vi "NI32LV90ASD1_DAQLinescan.vi"() -> ()   [LabVIEW 2009]
uses:
  ImageSettings.ctt
  DisplaySettings.ctt
  Instance          51 19Saved   DAQLinescan .vi
  Instance          52 19Saved   DAQLinescan .vi
  <vilib>/Utility/inputDevices.llb/mouseAcquire.vi
panel:
  in  "Laser 5":bool
  in  "Laser 8":bool
  in  "Laser 7":bool
  in  "Laser 6":bool
  out "Position":dbl[](array[numeric]) format="%.6f"
  in  "show position (PI digital)":bool
  in  "mouse wheel\nfocus control":bool
  out "mouse focus":cluster{"device ID":refnum<k1>, "Scrolling":i32}
  in  "Laser 4":bool
  in  "SyncTime(ns)":dbl=12.5
  in  "Laser 3":bool
  in  "Laser 2":bool
  in  "Laser 1":bool
  in  "AOTF":u16(ring) items=["None", "Laser 1", "Laser 2", "Laser 1 + 2", "Laser 3", "Laser 1 + 3", "Laser 2 + 3", "Laser 1+2+3", "Laser 1+2+3+4", "Laser 2+3+4"]
  in  "AOTF Setup":bool
  in  "x-scale: Time?":bool
  in  "Autoscale y-axis":bool=TRUE
  in  "Store Data":bool
  in  "Pick & Destroy":bool caption="stop"
  in  "Load Image":bool caption="stop"
  in  "Position Increment (µm)":cluster{"x":dbl, "y":dbl, "z":dbl}={"x"=0.1, "y"=0.1, "z"=0.1} {"z" format="%.2f"; "y" format="%.2f"; "x" format="%.2f"}
  in  "Current Position (µm)":cluster{"x":dbl, "y":dbl, "z":dbl} {"z" format="%.2f"; "y" format="%.2f"; "x" format="%.2f"}
  in  "Down (z)":bool
  in  "Up (z)":bool
  in  "Down":bool
  in  "Up":bool
  in  "Right":bool
  in  "Left":bool
  in  "Display Settings":T1={"Show MCS"=TRUE, "Show Image"=TRUE, "Color coding"=1, "Plane"=0, "Threshold"={"max"=150, "min"=0}} {"Plane" max=0; "Color coding" items=["Color Gradient", "False Color"]}
  in  "Destination:":path
  in  "Exit":bool caption="stop"
  in  "Save & Exit":bool caption="stop"
  in  "Stage Setup":bool
  in  "SPC Setup":bool
  in  "Scan":bool
  in  "EOM Setup":bool
  in  "Keep Start Position":bool=TRUE
  in  "Isotropy (x/y)":bool=TRUE
  in  "Keep Image Size":bool=TRUE
  in  "EOM":u16(ring) items=["None", "Trace", "Retrace", "All"]
  in  "Read Position":bool
  in  "Image Settings":T2={"Start Position (µm)"={"x"=0.0, "y"=0.0, "z"=0.0}, "End Position (µm)"={"x"=10.0, "y"=10.0, "z"=10.0}, "Image Resolution (nm/pixel)"={"x"=50.0, "y"=50.0, "z"=100.0}, "Image Size (µm)"={"x"=10.0, "y"=10.0, "z"=0.0}, "Image Size (pixel)"={"x"=200, "y"=200, "z"=0}, "Time Resolution\n(ms/pixel)"=1.0, "1st Axis"=0, "2nd Axis"=1, "Retrace"=FALSE, "Estimated Time"="00:00:40"} {"2nd Axis" items=["x", "y", "z"]; "1st Axis" items=["x", "y", "z"]; "Time Resolution\n(ms/pixel)" format="%.2f"; "Image Resolution (nm/pixel)"."z" format="%.2f"; "Image Resolution (nm/pixel)"."y" format="%.2f"; "Image Resolution (nm/pixel)"."x" format="%.2f"; "Image Size (µm)"."z" format="%.2f"; "Image Size (µm)"."y" format="%.2f"; "Image Size (µm)"."x" format="%.2f"; "End Position (µm)"."z" format="%.2f"; "End Position (µm)"."y" format="%.2f"; "End Position (µm)"."x" format="%.2f"; "Start Position (µm)"."z" format="%.2f"; "Start Position (µm)"."y" format="%.2f"; "Start Position (µm)"."x" format="%.2f"}
  out "MCS Trace":u32[][](graph)=[[5, 9, 9, 4, 5, 7, 7, 7, 4, 6, 5, 11, 11, 6, 8, 9, 8, 5, 6, 8, 5, 5, 8, 5, 6, 5, 4, 9, 6, 13, 5, 5, 6, 9, 9, 11, 9, 7, 5, 9, 10, 7, 6, 4, 9, 7, 8, 6, 9, 4, 7, 9, 3, 4, 6, 8, 5, 6, 5, 4, 6, 11, 8, 5, 9, 5, 8, 7, 8, 8, 7, 3, 5, 14, 7, 12, 10, 7, 8, 8, 7, 5, 6, 6, 6, 9, 9, 7, 8, 7, 9, 3, 11, 4, 8, 7, 4, 4, 4, 5, 6, 6, 12, 5, 8, 7, 8, 7, 5, 8, 10, 10, 9, 5, 7, 8, 4, 6, 9, 6, 8, 9, 9, 9, 3, 7, 4, 10, 8, 11, 8, 6, 7, 4, 6, 4, 11, 9, 11, 7, 8, 4, 6, 9, 11, 8, 11, 7, 6, 4, 13, 9, 5, 4, 8, 5, 11, 5, 6, 6, 6, 3, 8, 8, 8, 11, 8, 6, 5, 7, 10, 7, 10, 12, 6, 9, 7, 4, 8, 8, 9, 7, 6, 6, 5, 8, 8, 3, 10, 5, 5, 7, 9, 8, 14, 6, 9, 5, 8, 7], [0, 0, 0, 0, 0, 0, 0, 0, 0, 0, 0, 0, 0, 0, 0, 0, 0, 0, 0, 0, 0, 0, 0, 0, 0, 0, 0, 0, 0, 0, 0, 0, 0, 0, 0, 0, 0, 0, 0, 0, 0, 0, 0, 0, 0, 0, 0, 0, 0, 0, 0, 0, 0, 0, 0, 0, 0, 0, 0, 0, 0, 0, 0, 0, 0, 0, 0, 0, 0, 0, 0, 0, 0, 0, 0, 0, 0, 0, 0, 0, 0, 0, 0, 0, 0, 0, 0, 0, 0, 0, 0, 0, 0, 0, 0, 0, 0, 0, 0, 0, 0, 0, 0, 0, 0, 0, 0, 0, 0, 0, 0, 0, 0, 0, 0, 0, 0, 0, 0, 0, 0, 0, 0, 0, 0, 0, 0, 0, 0, 0, 0, 0, 0, 0, 0, 0, 0, 0, 0, 0, 0, 0, 0, 0, 0, 0, 0, 0, 0, 0, 0, 0, 0, 0, 0, 0, 0, 0, 0, 0, 0, 0, 0, 0, 0, 0, 0, 0, 0, 0, 0, 0, 0, 0, 0, 0, 0, 0, 0, 0, 0, 0, 0, 0, 0, 0, 0, 0, 0, 0, 0, 0, 0, 0, 0, 0, 0, 0, 0, 0], [0, 0, 0, 0, 0, 0, 0, 0, 0, 0, 0, 0, 0, 0, 0, 0, 0, 0, 0, 0, 0, 0, 0, 0, 0, 0, 0, 0, 0, 0, 0, 0, 0, 0, 0, 0, 0, 0, 0, 0, 0, 0, 0, 0, 0, 0, 0, 0, 0, 0, 0, 0, 0, 0, 0, 0, 0, 0, 0, 0, 0, 0, 0, 0, 0, 0, 0, 0, 0, 0, 0, 0, 0, 0, 0, 0, 0, 0, 0, 0, 0, 0, 0, 0, 0, 0, 0, 0, 0, 0, 0, 0, 0, 0, 0, 0, 0, 0, 0, 0, 0, 0, 0, 0, 0, 0, 0, 0, 0, 0, 0, 0, 0, 0, 0, 0, 0, 0, 0, 0, 0, 0, 0, 0, 0, 0, 0, 0, 0, 0, 0, 0, 0, 0, 0, 0, 0, 0, 0, 0, 0, 0, 0, 0, 0, 0, 0, 0, 0, 0, 0, 0, 0, 0, 0, 0, 0, 0, 0, 0, 0, 0, 0, 0, 0, 0, 0, 0, 0, 0, 0, 0, 0, 0, 0, 0, 0, 0, 0, 0, 0, 0, 0, 0, 0, 0, 0, 0, 0, 0, 0, 0, 0, 0, 0, 0, 0, 0, 0, 0]]
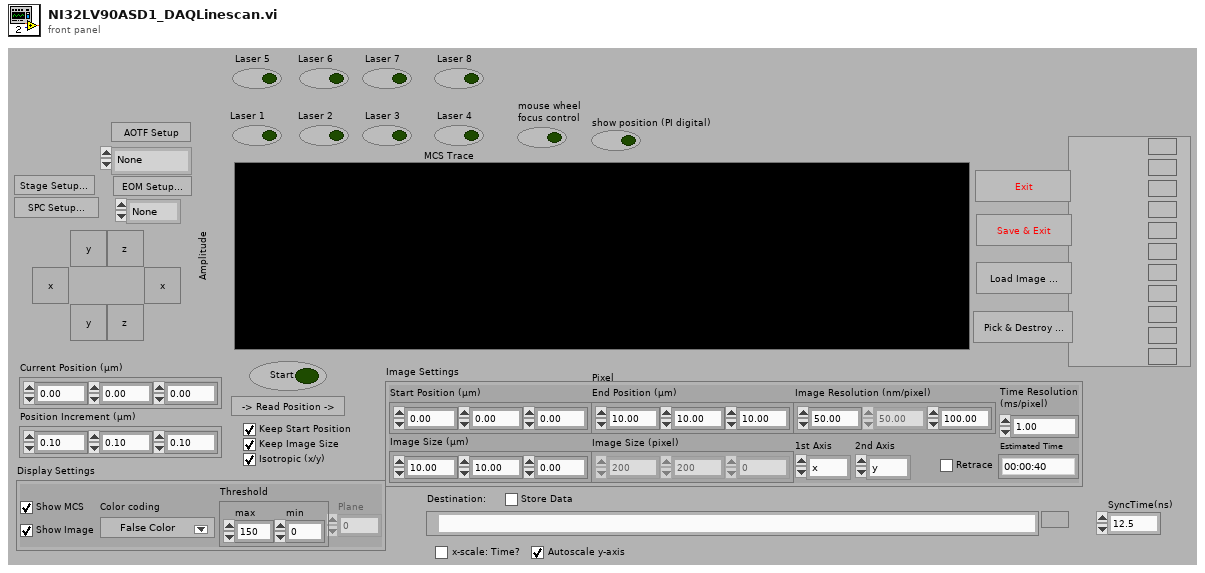
[diagram p1: front panel]
types:
  T1 = typedef "DisplaySettings.ctt" = cluster{"Show MCS":bool, "Show Image":bool, "Color coding":u16, "Plane":u32, "Threshold":cluster{"max":u32, "min":u32}}
  T2 = typedef "ImageSettings.ctt" = cluster{"Start Position (µm)":cluster{"x":dbl, "y":dbl, "z":dbl}, "End Position (µm)":cluster{"x":dbl, "y":dbl, "z":dbl}, "Image Resolution (nm/pixel)":cluster{"x":dbl, "y":dbl, "z":dbl}, "Image Size (µm)":cluster{"x":dbl, "y":dbl, "z":dbl}, "Image Size (pixel)":cluster{"x":u32, "y":u32, "z":u32}, "Time Resolution\n(ms/pixel)":dbl, "1st Axis":u16, "2nd Axis":u16, "Retrace":bool, "Estimated Time":string}
  T3 = enum16{"Get Type", "Set Type", "GetStageInit", "GetWriteStageSetting", "GetInitializeStageOutput", "GetSetAxisPosition", "GetSetPos", "GetSetupStage", "HaltStageOutput"}
  T4 = enum16{"Get Type", "Set Type", "GetStageInit", "GetWriteStageSetting", "GetInitializeStageOutput", "GetSetAxisPosition", "GetSetPos"}
  T5 = typedef "FIFOSettings.ctt" = cluster{"Measurement":cluster{"Binning (ms)":sgl, "External Trigger Condition":u16, "Stop Condition:":u16, "Stop Count":dbl, "Buffer Size (Photons)":u32, "No of Channels":u16, "Ext Latch Delay":i16}, "ADC":cluster{"Binning (HH)":i16, "Dither Range":i16, "Count Increment":i16, "Mode":u16}, "SYNC":cluster{"SYNC ZC Level (mV)":sgl, "SYNC Freq Divider":u16, "SYNC Holdoff (ps)":sgl, "SYNC Threshold (mV)":sgl}, "TAC":cluster{"TAC Range (ns)":sgl, "TAC Gain":i16, "TAC Offset (%)":sgl, "TAC Limit Low (%)":sgl, "TAC Limit High (%)":sgl}, "Ch 2":cluster{"Ch2 ZC Level (mV)":sgl, "Ch2 Holdoff (ps)":sgl, "Ch2 Threshold (mV)":sgl}, "Ch 3":cluster{"Ch3 ZC Level (mV)":sgl, "Ch3 Holdoff (ps)":sgl, "Ch3 Threshold (mV)":sgl}, "Ch 4":cluster{"Ch4 ZC Level (mV)":sgl, "Ch4 Holdoff (ps)":sgl, "Ch4 Threshold (mV)":sgl}, "Ch1":cluster{"Ch1 ZC Level (mV)":sgl, "Ch1 Holdoff (ps)":sgl, "Ch1 Threshold (mV)":sgl}}
  T6 = typedef "DAQLinescanVisualization.ctt" = cluster{"Threshold":u32, "Trace Window #":u32, "IMAQ Trace":T7, "Retrace Window #":u32, "IMAQ Retrace":T7}
  T7 = typedef "IMAQ Image.ctl" = refnum<image>
  T8 = typedef "LineScanStatus.ctt" = cluster{"in line":bool, "line status":cluster{"count":u32, "current":cluster{"x":u32, "y":u32, "z":u32}}, "plane status":cluster{"count":u32, "current":cluster{"x":u32, "y":u32, "z":u32}}, "new line step":cluster{"x":dbl, "y":dbl, "z":dbl}, "new plane step":cluster{"x":dbl, "y":dbl, "z":dbl}}
  T9 = typedef "StageType.ctt" = enum16{"PI 725 USB", "PI 725 TCP/IP", "PI analogue step"}
  T10 = cluster{"Start Position (µm)":cluster{"x":dbl, "y":dbl, "z":dbl}, "End Position (µm)":cluster{"x":dbl, "y":dbl, "z":dbl}, "Image Resolution (nm/pixel)":cluster{"x":dbl, "y":dbl, "z":dbl}, "Image Size (µm)":cluster{"x":dbl, "y":dbl, "z":dbl}, "Image Size (pixel)":cluster{"x":u32, "y":u32, "z":u32}, "Time Resolution\n(ms/pixel)":dbl, "1st Axis":u16, "2nd Axis":u16, "Retrace":bool, "Estimated Time":string}
  T11 = typedef "ScannedImage.ctl" = cluster{"BinningMicroS":dbl, "OverflowConstant":dbl, "MacrotimeCycle":dbl, "Trace":u32[][][][], "Retrace":u32[][][][], "current line":i32, "current plane":i32}
  T12 = cluster{"Horizontal":i32, "Vertical":i32, "Scrolling":i32}
  T13 = typedef "LVMinMaxIncTypeDef.ctl" = cluster{"Minimum":dbl, "Maximum":dbl, "Increment":dbl}
  T14 = typedef "AnalogSettings.ctt" = cluster{"PCI 671x Device Number":u32, "Samples per Unit":u32}
  T15 = typedef "AOTFSettings.ctt" = cluster{"Laser 1 Output Channel":tag, "AOTF  1 Output Voltage":dbl, "Laser 2 Output Channel":tag, "AOTF  2 Output Voltage":dbl, "Laser 3 Output Channel":tag, "AOTF  3 Output Voltage":dbl, "Pixel per Cycle":u16, "Time per Cycle  / ms":dbl, "Laser 4 Output Channel":tag, "AOTF  4 Output Voltage":dbl, "Laser 5 Output Channel":tag, "AOTF 5 Output Voltage ":dbl, "Laser 6 Output Channel":tag, "AOTF  6 Output Voltage ":dbl, "Laser 7 Output Channel":tag, "AOTF 7 Output Voltage ":dbl, "Laser 8 Output Channel":tag, "AOTF  8 Output Voltage ":dbl, "AOTF  1 Frequency":dbl, "AOTF  2 Frequency":dbl, "AOTF  3  Frequency":dbl, "AOTF  4 Frequency":dbl, "AOTF 5 Frequency":dbl, "AOTF  6 Frequency":dbl, "AOTF 7  Frequency":dbl, "AOTF  8 Frequency":dbl, "AOTF  1 Amplitude":dbl, "AOTF  2 Amplitude":dbl, "AOTF  3  Amplitude":dbl, "AOTF  4 Amplitude":dbl, "AOTF 5 Amplitude":dbl, "AOTF  6 Amplitude":dbl, "AOTF 7 Amplitude  ":dbl, "AOTF  8 Amplitude":dbl}
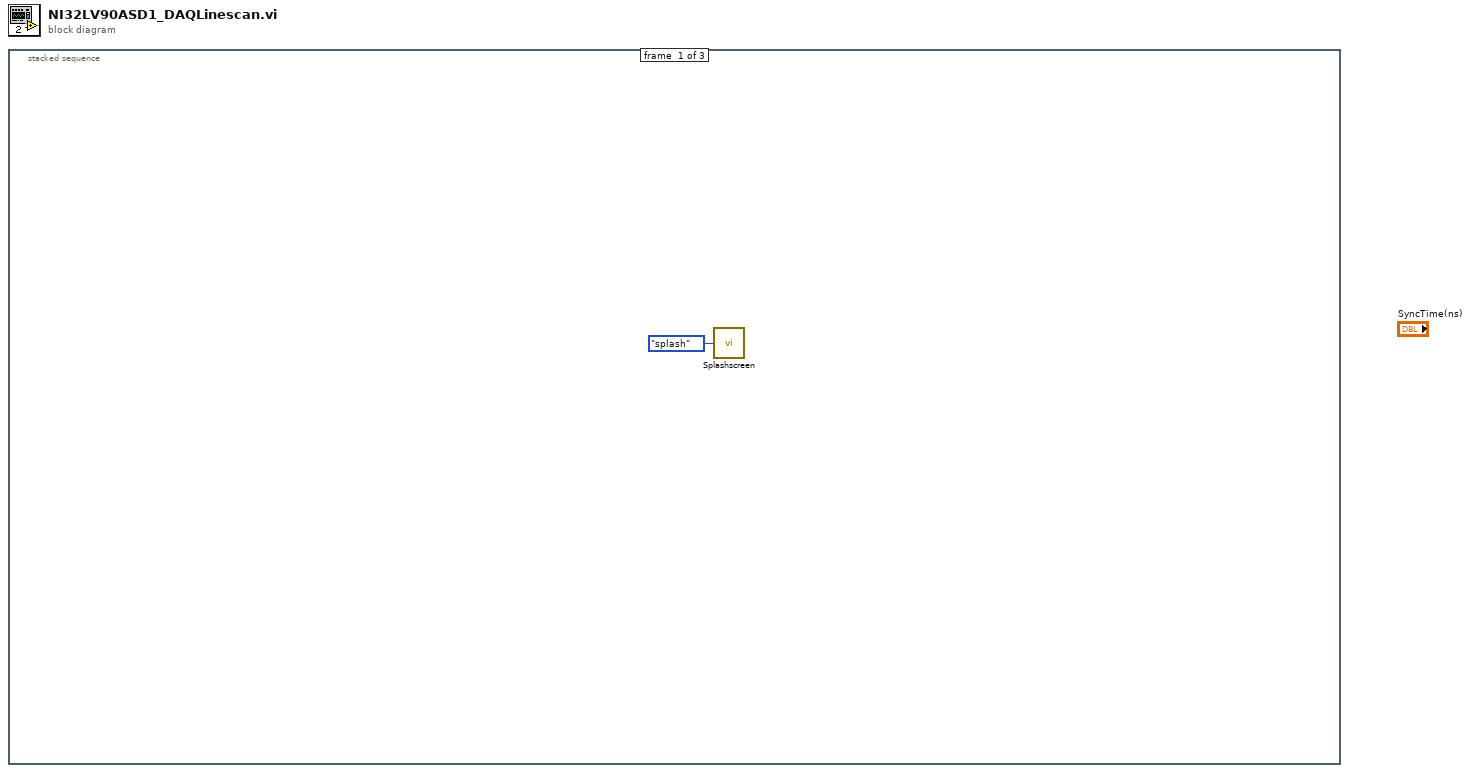
[diagram p0: block diagram]
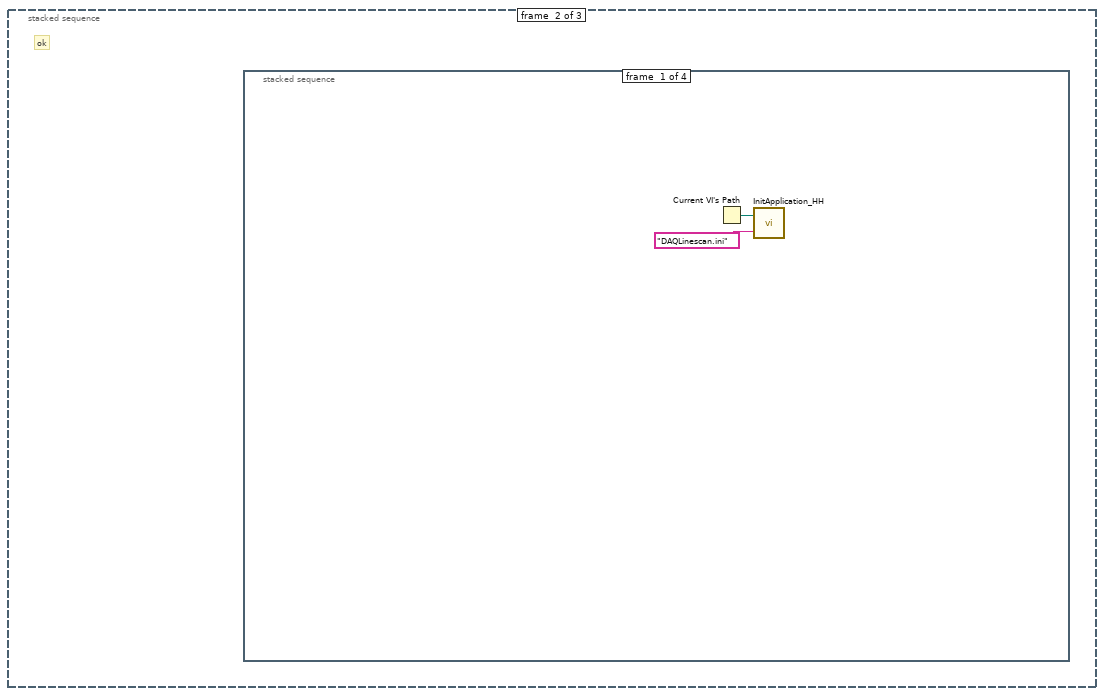
[diagram p2: hidden frame]
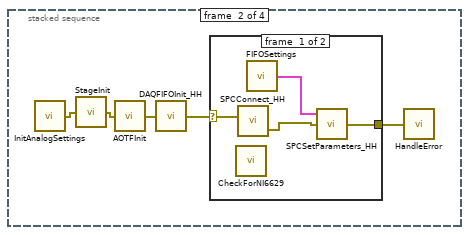
[diagram p3: hidden frame]
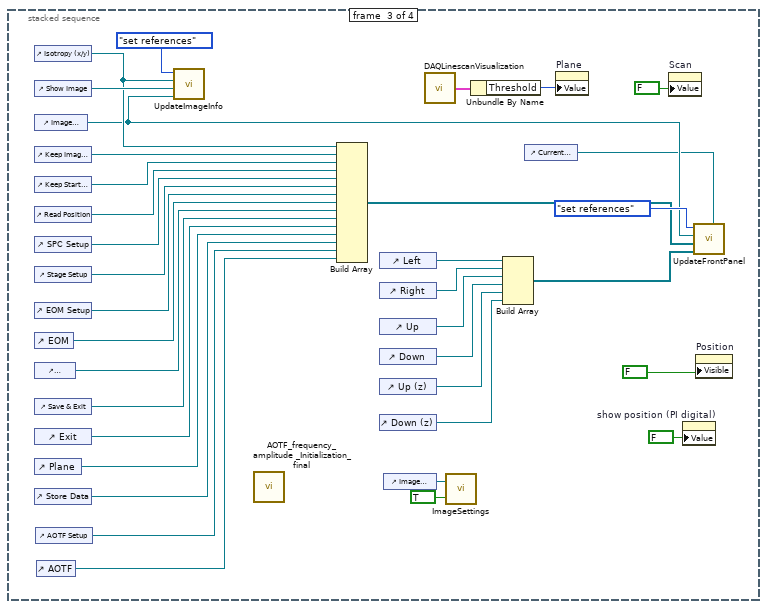
[diagram p5: hidden frame]
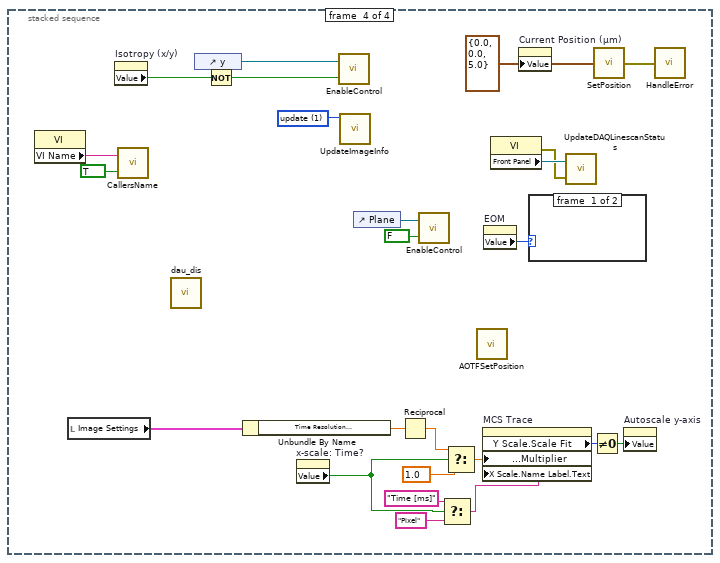
[diagram p6: hidden frame]
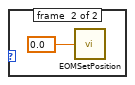
[diagram p7: hidden frame]
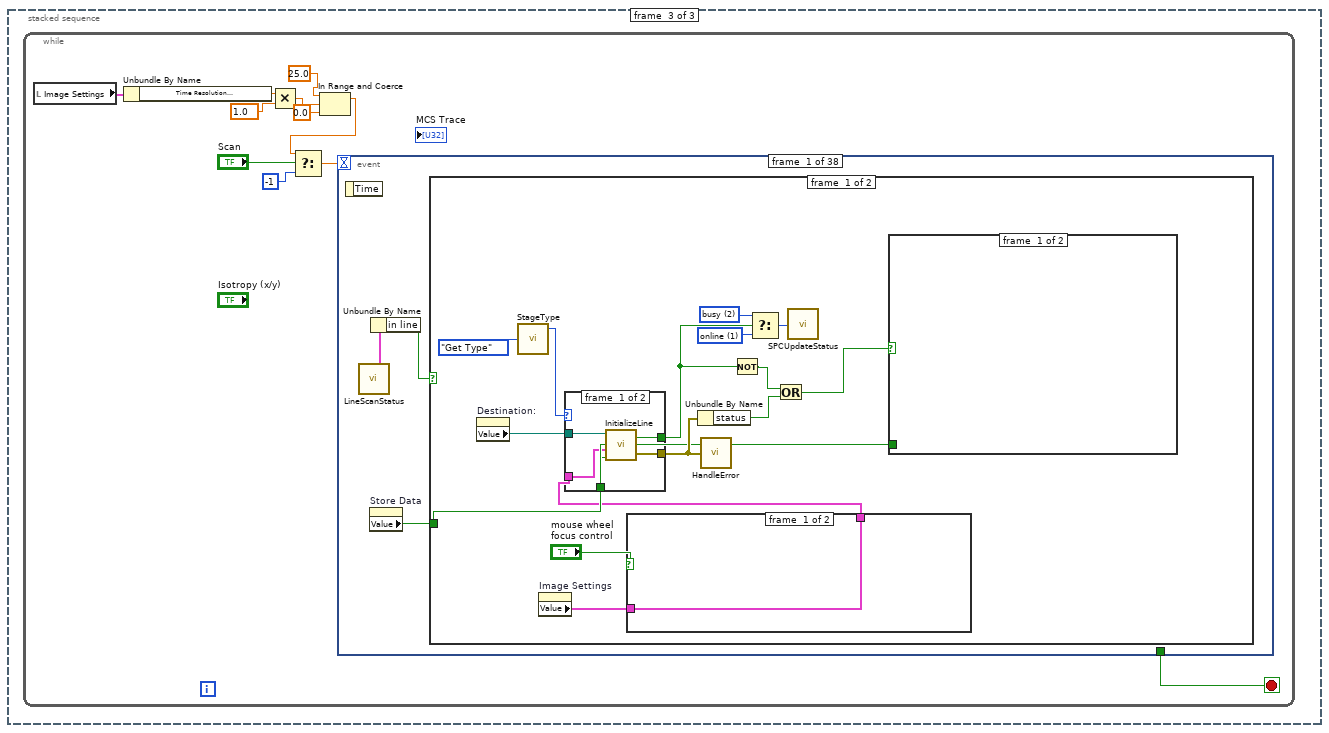
[diagram p8: hidden frame]
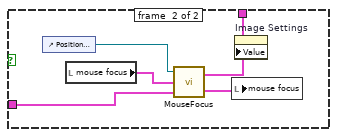
[diagram p9: hidden frame]
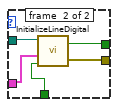
[diagram p10: hidden frame]
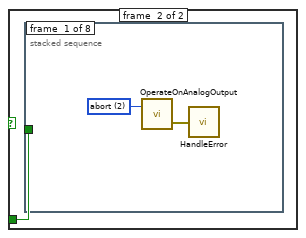
[diagram p11: hidden frame]
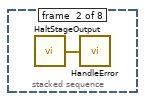
[diagram p12: hidden frame]
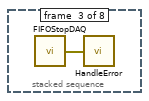
[diagram p13: hidden frame]
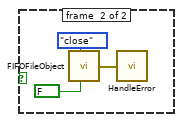
[diagram p15: hidden frame]
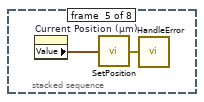
[diagram p16: hidden frame]
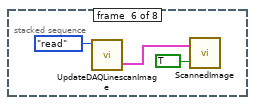
[diagram p17: hidden frame]
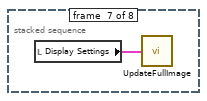
[diagram p18: hidden frame]
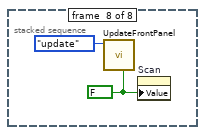
[diagram p19: hidden frame]
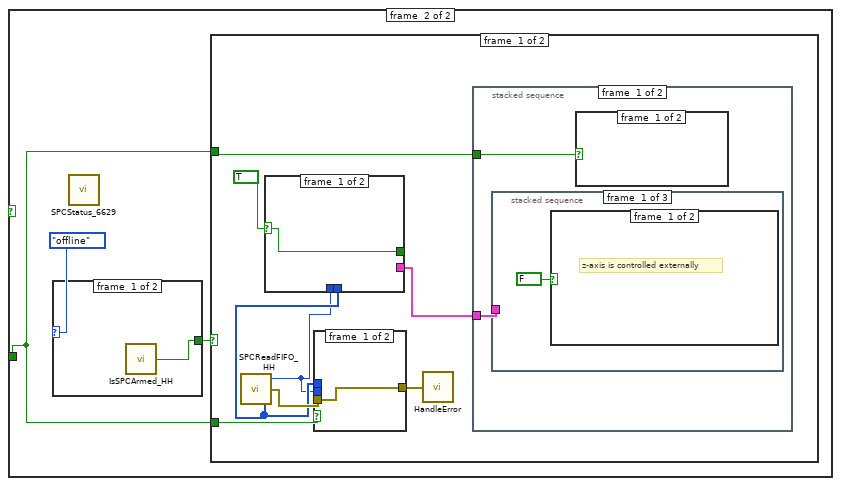
[diagram p20: hidden frame]
diagram:
  n1 = stacked-sequence {
    frame #0 {
      n2 = call "Splashscreen.vi"("Mode"=enum16{"splash", "dialog"}."splash") -> ()  [unwired: 1 in]
    }
    frame #1 {
      # "ok"
      n3 = stacked-sequence {
        frame #0 {
          n4 = Current VI's Path() -> (path=w3:path)
          n5 = call "InitApplication_HH.vi"("file name"="DAQLinescan.ini", "VI path"=w3) -> ()
        }
        frame #1 {
          n6 = call "InitAnalogSettings.vi"() -> ("error out"=w5:errorcluster)  [unwired: 1 in]
          n7 = call "StageInit.vi"("error in (no error)"=w5) -> ("error out"=w4:errorcluster)
          n8 = call "AOTFInit.vi"("error in (no error)"=w4) -> ("error out"=w6:errorcluster)
          n9 = call "DAQFIFOInit_HH.vi"("error in (no error)"=w6) -> ("error out"=w8:errorcluster)
          n10 = case shown="No Error" w8 {
            selector: w8 -> [w10 w13]
            tunnel: [w11 w13] -> w7
            frame #0 {
              n11 = call "CheckForNI6629.vi"() -> ()  [unwired: 1 in]
              n12 = call "SPCConnect_HH.vi"("error in (no error)"=w10) -> ("Error out"=w9:errorcluster)  [unwired: 1 in]
              n13 = call "FIFOSettings.vi"() -> ("FIFO Settings(out)"=w12:T5)  [unwired: 2 in]
              n14 = call "SPCSetParameters_HH.vi"("error in (no error)"=w9, "FIFO Settings"=w12) -> ("error (out)"=w11:errorcluster)  [unwired: 1 in]
            }
            frame #1 {
            }
          }
          n15 = call "HandleError.vi"("error in (no error)"=w7) -> ()
        }
        frame #2 {
          n16 = control-ref of="Isotropy (x/y)"() -> (w27:refnum<vi>)
          n17 = control-ref of="Show Image"() -> (w46:refnum<vi>)
          n18 = control-ref of="Image Settings"() -> (w26:refnum<vi>)
          n19 = control-ref of="Keep Image Size"() -> (w45:refnum<vi>)
          n20 = control-ref of="Keep Start Position"() -> (w44:refnum<vi>)
          n21 = control-ref of="Read Position"() -> (w43:refnum<vi>)
          n22 = control-ref of="SPC Setup"() -> (w42:refnum<vi>)
          n23 = control-ref of="Stage Setup"() -> (w41:refnum<vi>)
          n24 = control-ref of="EOM Setup"() -> (w40:refnum<vi>)
          n25 = control-ref of="EOM"() -> (w39:refnum<vi>)
          n26 = control-ref of="Destination:"() -> (w38:refnum<vi>)
          n27 = control-ref of="Save & Exit"() -> (w37:refnum<vi>)
          n28 = control-ref of="Exit"() -> (w36:refnum<vi>)
          n29 = control-ref of="Plane"() -> (w22:refnum<vi>)
          n30 = control-ref of="Store Data"() -> (w21:refnum<vi>)
          n31 = control-ref of="AOTF Setup"() -> (w17:refnum<vi>)
          n32 = control-ref of="AOTF"() -> (w16:refnum<vi>)
          n33 = call "UpdateImageInfo.vi"("Image Refnum"=w26, "Show Image Refnum"=w46, "Isotropy (x/y) Refnum"=w27, "operation"=enum16{"set references", "update"}."set references") -> ()
          n34 = call "AOTF_frequency_amplitude _Initialization_final.vi"() -> ()  [unwired: 1 in]
          n35 = Build Array(w27, w45, w44, w43, w42, w41, w40, w39, w38, w37, w36, w22, w21, w17, w16) -> (w25:refnum<vi>[])
          n36 = control-ref of="Left"() -> (w35:refnum<vi>)
          n37 = control-ref of="Right"() -> (w34:refnum<vi>)
          n38 = control-ref of="Up"() -> (w33:refnum<vi>)
          n39 = control-ref of="Down"() -> (w32:refnum<vi>)
          n40 = control-ref of="Up (z)"() -> (w31:refnum<vi>)
          n41 = control-ref of="Down (z)"() -> (w30:refnum<vi>)
          n42 = control-ref of="Image Settings"() -> (w19:refnum<vi>)
          n43 = call "DAQLinescanVisualization.vi"() -> ("Visualization (output)"=w47:T6)  [unwired: 2 in]
          n44 = call "ImageSettings.vi"("set"=TRUE ("s"), "Image Settings in"=w19) -> ()  [unwired: 1 out]
          n45 = Unbundle By Name(w47) -> ("Threshold"=w48:u32)
          n46 = Build Array(w35, w34, w33, w32, w31, w30) -> (w24:refnum<vi>[])
          n47 = control-ref of="Current Position (µm)"() -> (w23:refnum<vi>)
          n48 = property on="Plane" class="DigNum (strict)"("Value"=w48) -> ()  [unwired: 2 in, 2 out]
          n49 = property on="Scan" class="Bool (strict)"("Value"=FALSE ("Scan")) -> ()  [unwired: 2 in, 2 out]
          n50 = property on="show position (PI digital)" class="Bool (strict)"("Value"=FALSE ("show position (PI digital)")) -> ()  [unwired: 2 in, 2 out]
          n51 = call "UpdateFrontPanel.vi"("operation"=enum16{"set references", "update"}."set references", "Image Settings"=w26, "Regular Controls"=w25, "Special Controls"=w24, "Current Position (µm)"=w23) -> ()  [unwired: 5 in]
          n52 = property on="Position" class="Arr (strict)"("Visible"=FALSE) -> ()  [unwired: 2 in, 2 out]
        }
        frame #3 {
          w66 = u16 1 items=["set references", "update"] ("operation")
          w70 = cluster{"x":dbl, "y":dbl, "z":dbl} {"x"=0.0, "y"=0.0, "z"=5.0} ("Current Position (µm)")
          n53 = property class="VI"() -> ("VI Name"=w61:string)  [unwired: 2 in, 2 out]
          n54 = local read "Image Settings"() -> (w57:T2)
          n55 = property on="Isotropy (x/y)" class="Boolean (strict)"() -> ("Value"=w67:bool)  [unwired: 2 in, 2 out]
          n56 = call "CallersName.vi"("Get/Set"=TRUE ("s"), "Callers Name"=w61) -> ()  [unwired: 1 out]
          n57 = call "dau_dis.vi"() -> ()  [unwired: 1 in]
          n58 = control-ref of="y"() -> (w72:refnum<vi>)
          n59 = Not(x=w67) -> (.not. x?=w71:bool)
          n60 = Unbundle By Name(w57) -> ("Time Resolution\n(ms/pixel)"=w56:dbl)
          n61 = property on="x-scale: Time?" class="Boolean (strict)"() -> ("Value"=w50:bool)  [unwired: 2 in, 2 out]
          n62 = call "EnableControl.vi"("Enable"=w71, "Reference"=w72) -> ()
          n63 = call "UpdateImageInfo.vi"("operation"=w66) -> ()  [unwired: 3 in]
          n64 = control-ref of="Plane"() -> (w65:refnum<vi>)
          n65 = Reciprocal(x=w56) -> (1/x=w54:dbl)
          n66 = call "EnableControl.vi"("Enable"=FALSE, "Reference"=w65) -> ()
          n67 = Select(t="Time [ms]", s=w50, f="Pixel") -> (s? t:f=w49:string)
          n68 = Select(t=w54, s=w50, f=1.0) -> (s? t:f=w55:dbl)
          n69 = call "AOTFSetPosition.vi"() -> ()  [unwired: 2 in]
          n70 = property on="MCS Trace" class="WaveformChart (strict)"("X Scale.Offset and Multiplier:Multiplier"=w55, "X Scale.Name Label.Text"=w49) -> ("Y Scale.Scale Fit"=w59:u8)  [unwired: 2 in, 2 out]
          n71 = property on="EOM" class="Ring (strict)"() -> ("Value"=w62:u16)  [unwired: 2 in, 2 out]
          n72 = property class="VI"() -> (error out=w68:errorcluster, "Front Panel"=w69:refnum<vi>)  [unwired: 2 in, 1 out]
          n73 = property on="Current Position (µm)" class="Cluster (strict)"("Value"=w70) -> ()  [unwired: 2 in, 2 out]
          n74 = case shown="0" w62 {
            frame #0 {
            }
            frame #1 {
              n75 = call "EOMSetPosition.vi"("value"=sgl 0.0) -> ()
            }
          }
          n76 = call "UpdateDAQLinescanStatus.vi"("error in (no error)"=w68, "Panel"=w69) -> ()
          n77 = Not Equal To 0?(x=w59) -> (x != 0?=w58:bool)
          n78 = call "SetPosition.vi"("Current Position (µm)"=w70) -> ("error out"=w63:errorcluster)
          n79 = property on="Autoscale y-axis" class="Bool (strict)"("Value"=w58) -> ()  [unwired: 2 in, 2 out]
          n80 = call "HandleError.vi"("error in (no error)"=w63) -> ()
        }
      }
    }
    frame #2 {
      n81 = while {
        stop <- w80 stop-if-true
        n82 = local read "Image Settings"() -> (w81:T2)
        n83 = Unbundle By Name(w81) -> ("Time Resolution\n(ms/pixel)"=w79:dbl)
        n84 = Multiply(x=w79, y=1.0) -> (x*y=w77:dbl)
        n85 = In Range and Coerce(upper limit=25.0, x=w77, lower limit=0.0) -> (coerced(x)=w74:dbl)  [unwired: 1 out]
        n86 = Select(t=w74, s="Scan", f=-1) -> (s? t:f=w84:dbl)
        n87 = event shown="[28] \"Pick & Destroy\": Value Change" {
          selector: _ -> [_ _ _ _ _ _ _ _ _ _ _ _ _ _ _ _ _ _ _ _ _ _ _ _ _ _ _ _ _ _ _ _ _ _ _ _ _ _]
          dyn-events: _ -> [_ _ _ _ _ _ _ _ _ _ _ _ _ _ _ _ _ _ _ _ _ _ _ _ _ _ _ _ _ _ _ _ _ _ _ _ _ _]
          timeout: w84 -> [_ _ _ _ _ _ _ _ _ _ _ _ _ _ _ _ _ _ _ _ _ _ _ _ _ _ _ _ _ _ _ _ _ _ _ _ _ _]
          tunnel: [_ _ _ _ _ _ _ _ _ _ _ _ _ _ _ _ _ _ _ _ _ _ _ _ _ TRUE _ _ _ _ _ _ _ _ _ _ _ _] -> w80
          event #0 {
            n88 = event-data() -> ()  [unwired: 1 in, 1 out]
            n89 = call "LineScanStatus.vi"() -> ("Linescan Status (output)"=w86:T8)  [unwired: 2 in]
            n90 = property on="Store Data" class="Boolean (strict)"() -> ("Value"=w85:bool)  [unwired: 2 in, 2 out]
            n91 = Unbundle By Name(w86) -> ("in line"=w87:bool)
            n92 = case shown="True" w87 {
              tunnel: w85 -> [w93 w138]
              frame #0 {
                w100 = u16 1 items=["offline", "online", "busy"] ("Status (input)")
                w101 = u16 2 items=["offline", "online", "busy"] ("Status (input)")
                n93 = property on="Destination:" class="Path"() -> ("Value"=w102:path)  [unwired: 2 in, 2 out]
                n94 = call "StageType.vi"("Function"=T3."Get Type") -> ("Stage Type (output)"=w91:T9)  [unwired: 2 in, 2 out]
                n95 = property on="Image Settings" class="Cluster (strict)"() -> ("Value"=w90:T10)  [unwired: 2 in, 2 out]
                n96 = case shown="False" "mouse wheel\nfocus control" {
                  tunnel: w90 -> [w103 w108]
                  tunnel: [w103 w107] -> w89
                  frame #0 {
                  }
                  frame #1 {
                    n97 = control-ref of="Position Increment (µm)"() -> (w104:refnum<vi>)
                    n98 = local read "mouse focus"() -> (w106:cluster{"device ID":refnum<k1>, "Scrolling":i32})
                    n99 = call "MouseFocus.vi"("Image Settings"=w108, "mouse focus"=w106, "Position increment"=w104) -> ("mouse focus"=w105:cluster{"device ID":refnum<k1>, "Scrolling":i32}, "Image Settings"=w107:T10)
                    n100 = local write "mouse focus"(w105) -> ()
                    n101 = property on="Image Settings" class="Clust (strict)"("Value"=w107) -> ()  [unwired: 2 in, 2 out]
                  }
                }
                n102 = case shown="\"PI 725 USB\", \"PI 725 TCP/IP\"" w91 {
                  tunnel: w102 -> [w113 w118]
                  tunnel: w89 -> [w112 w117]
                  tunnel: [w111 w115] -> w98
                  tunnel: [w110 w114] -> w97
                  tunnel: w93 -> [w109 w116]
                  frame #0 {
                    n103 = call "InitializeLine.vi"("Store Data"=w109, "Image Settings"=w112, "Destination:"=w113) -> ("error out"=w111:errorcluster, "Busy"=w110:bool)  [unwired: 1 in]
                  }
                  frame #1 {
                    n104 = call "InitializeLineDigital.vi"("Store Data"=w116, "Image Settings"=w117, "Destination:"=w118) -> ("error out"=w115:errorcluster, "Busy"=w114:bool)  [unwired: 1 in]
                  }
                }
                n105 = Unbundle By Name(w98) -> ("status"=w95:bool)
                n106 = call "HandleError.vi"("error in (no error)"=w98) -> ()
                n107 = Not(x=w97) -> (.not. x?=w96:bool)
                n108 = Select(t=w101, s=w97, f=w100) -> (s? t:f=w99:u16)
                n109 = Or(x=w96, y=w95) -> (x .or. y?=w94:bool)
                n110 = call "SPCUpdateStatus.vi"("Status"=w99) -> ()
                n111 = case shown="True" w94 {
                  tunnel: w93 -> [_ w119]
                  frame #0 {
                  }
                  frame #1 {
                    n112 = stacked-sequence {
                      tunnel: w119 -> [_ _ _ w124 _ _ _ _]
                      frame #0 {
                        w121 = u16 2 items=["start", "state", "abort"] ("operation")
                        n113 = call "OperateOnAnalogOutput.vi"("operation"=w121) -> ("error out"=w120:errorcluster)  [unwired: 1 in, 1 out]
                        n114 = call "HandleError.vi"("error in (no error)"=w120) -> ()
                      }
                      frame #1 {
                        n115 = call "HaltStageOutput.vi"() -> ("Error out"=w122:errorcluster)  [unwired: 1 in]
                        n116 = call "HandleError.vi"("error in (no error)"=w122) -> ()
                      }
                      frame #2 {
                        n117 = call "FIFOStopDAQ.vi"() -> ("error out"=w123:errorcluster)
                        n118 = call "HandleError.vi"("error in (no error)"=w123) -> ()
                      }
                      frame #3 {
                        n119 = case shown="True" w124 {
                          frame #0 {
                          }
                          frame #1 {
                            n120 = call "FIFOFileObject.vi"(".sm file format"=FALSE, "function (open:0)"=enum16{"open", "write", "close"}."close") -> ("error out"=w126:errorcluster)  [unwired: 4 in]
                            n121 = call "HandleError.vi"("error in (no error)"=w126) -> ()
                          }
                        }
                      }
                      frame #4 {
                        n122 = property on="Current Position (µm)" class="Cluster (strict)"() -> ("Value"=w129:cluster{"x":dbl, "y":dbl, "z":dbl})  [unwired: 2 in, 2 out]
                        n123 = call "SetPosition.vi"("Current Position (µm)"=w129) -> ("error out"=w128:errorcluster)
                        n124 = call "HandleError.vi"("error in (no error)"=w128) -> ()
                      }
                      frame #5 {
                        n125 = call "UpdateDAQLinescanImage.vi"("operation"=enum16{"initialize", "update", "read"}."read") -> ("LinescanSampling"=w132:T11)  [unwired: 3 in, 1 out]
                        n126 = call "ScannedImage.vi"("Get/Set"=TRUE, "Scanned Image (input)"=w132) -> ()  [unwired: 1 out]
                      }
                      frame #6 {
                        n127 = local read "Display Settings"() -> (w133:T1)
                        n128 = call "UpdateFullImage.vi"("Display Settings"=w133) -> ()
                      }
                      frame #7 {
                        w135 = FALSE ("Scan")
                        n129 = call "UpdateFrontPanel.vi"("operation"=enum16{"set references", "update"}."update", "Scan"=w135) -> ()  [unwired: 8 in]
                        n130 = property on="Scan" class="Boolean (strict)"("Value"=w135) -> ()  [unwired: 2 in, 2 out]
                      }
                    }
                  }
                }
              }
              frame #1 {
                n131 = case shown="\"offline\", Default" enum16{"offline", "online", "busy"}."offline" ("Status (output)") {
                  tunnel: [w139 FALSE] -> w137
                  frame #0 {
                    n132 = call "IsSPCArmed_HH.vi"() -> ("Boolean"=w139:bool)  [unwired: 1 in]
                  }
                  frame #1 {
                  }
                }
                n133 = call "SPCStatus_6629.vi"() -> ()  [unwired: 2 in, 1 out]
                n134 = case shown="True" w137 {
                  tunnel: w138 -> [w141 w186]
                  tunnel: w138 -> [w143 w185]
                  frame #0 {
                    n135 = call "SPCReadFIFO_HH.vi"() -> ("count"=w144:i32, "error out"=w148:errorcluster, "buffer"=w146:u32[])  [unwired: 2 in]
                    n136 = case shown="True" TRUE ("Case Constant\n(See Context Help) 2") {
                      selector: TRUE ("Case Constant\n(See Context Help) 2") -> [w169 _]
                      tunnel: w144 -> [_ w174]
                      tunnel: w146 -> [_ w173]
                      tunnel: [w169 w172] -> _
                      tunnel: [_ w171] -> w142
                      frame #0 {
                      }
                      frame #1 {
                        n137 = call "UpdateDAQLinescanImage.vi"("buffer (output)"=w173, "count (read)"=w174, "operation"=enum16{"initialize", "update", "read"}."update") -> ("LinescanSampling"=w171:T11, "end of line"=w172:bool)  [unwired: 1 in]
                      }
                    }
                    n138 = case shown="True" w143 {
                      tunnel: w148 -> [w175 w180]
                      tunnel: [w175 w179] -> w147
                      tunnel: w144 -> [_ w178]
                      tunnel: w146 -> [_ w177]
                      frame #0 {
                      }
                      frame #1 {
                        n139 = call "FIFOFileObject.vi"(".sm file format"=FALSE, "function (open:0)"=enum16{"open", "write", "close"}."write", "error in (no error)"=w180, "count"=w178, "buffer"=w177) -> ("error out"=w179:errorcluster)  [unwired: 1 in]
                      }
                    }
                    n140 = call "HandleError.vi"("error in (no error)"=w147) -> ()
                    n141 = stacked-sequence {
                      tunnel: w142 -> [w150 _]
                      tunnel: w141 -> [w149 _]
                      frame #0 {
                        n142 = stacked-sequence {
                          tunnel: w150 -> [_ _ w160]
                          frame #0 {
                            n143 = case shown="False" FALSE {
                              frame #0 {
                                # "z-axis is controlled externally"
                              }
                              frame #1 {
                                w153 = 2
                                # "third axis"
                                n144 = property on="Current Position (µm)" class="Clust (strict)"() -> ("Value"=w152:cluster{"x":dbl, "y":dbl, "z":dbl})  [unwired: 2 in, 2 out]
                                n145 = Cluster To Array(cluster=w152) -> (array=w154:dbl[])
                                n146 = Index Array(array=w154, index=w153) -> (element=w155:dbl)
                                n147 = call "SetAxisPos.vi"("Position"=w155, "Axis"=w153) -> ("error out"=w156:errorcluster)
                                n148 = call "HandleError.vi"("error in (no error)"=w156) -> ()
                              }
                            }
                          }
                          frame #1 {
                            n149 = call "HaltStageOutput.vi"() -> ("Error out"=w157:errorcluster)  [unwired: 1 in]
                            n150 = call "HandleError.vi"("error in (no error)"=w157) -> ()
                          }
                          frame #2 {
                            n151 = call "FIFOStopDAQ.vi"() -> ("error out"=w161:errorcluster)
                            n152 = call "HandleError.vi"("error in (no error)"=w161) -> ()
                            n153 = call "OperateOnAnalogOutput.vi"("operation"=enum16{"start", "state", "abort"}."abort") -> ("error out"=w162:errorcluster)  [unwired: 1 in, 1 out]
                            n154 = call "UpdateDAQLinescanDisplay.vi"("LinescanSampling"=w160, "operation"=enum16{"initialize", "update"}."update") -> ()  [unwired: 3 in]
                            n155 = call "HandleError.vi"("error in (no error)"=w162) -> ()
                          }
                        }
                        n156 = case shown="True" w149 {
                          frame #0 {
                          }
                          frame #1 {
                            n157 = call "FIFOFileObject.vi"(".sm file format"=FALSE, "function (open:0)"=enum16{"open", "write", "close"}."close") -> ("error out"=w164:errorcluster)  [unwired: 4 in]
                            n158 = call "HandleError.vi"("error in (no error)"=w164) -> ()
                          }
                        }
                      }
                      frame #1 {
                        n159 = local read "Image Settings"() -> (w166:T2)
                        n160 = call "NextLine.vi"("Image Settings"=w166) -> ("Continue Scan"=w167:bool)
                        n161 = case shown="True" w167 {
                          frame #0 {
                          }
                          frame #1 {
                          }
                        }
                        n162 = call "UpdateFrontPanel.vi"("operation"=enum16{"set references", "update"}."update", "Scan"=w167) -> ()  [unwired: 8 in]
                        n163 = property on="Scan" class="Bool (strict)"("Value"=w167) -> ()  [unwired: 2 in, 2 out]
                      }
                    }
                  }
                  frame #1 {
                    n164 = call "SPCReadFIFO_HH.vi"() -> ("count"=w182:i32, "error out"=w190:errorcluster, "buffer"=w188:u32[])  [unwired: 2 in]
                    n165 = case shown="True" TRUE ("Case Constant\n(See Context Help) 2") {
                      selector: TRUE ("Case Constant\n(See Context Help) 2") -> [w191 _]
                      tunnel: w182 -> [_ w196]
                      tunnel: w188 -> [_ w195]
                      tunnel: [w191 w194] -> w183
                      tunnel: [_ w193] -> w187
                      frame #0 {
                      }
                      frame #1 {
                        n166 = call "UpdateDAQLinescanImage.vi"("buffer (output)"=w195, "count (read)"=w196, "operation"=enum16{"initialize", "update", "read"}."update") -> ("LinescanSampling"=w193:T11, "end of line"=w194:bool)  [unwired: 1 in]
                      }
                    }
                    n167 = case shown="False" w185 {
                      tunnel: w190 -> [w197 w202]
                      tunnel: [w197 w201] -> w189
                      tunnel: w182 -> [_ w200]
                      tunnel: w188 -> [_ w199]
                      frame #0 {
                      }
                      frame #1 {
                        n168 = call "FIFOFileObject.vi"(".sm file format"=FALSE, "function (open:0)"=enum16{"open", "write", "close"}."write", "error in (no error)"=w202, "count"=w200, "buffer"=w199) -> ("error out"=w201:errorcluster)  [unwired: 1 in]
                      }
                    }
                    n169 = call "HandleError.vi"("error in (no error)"=w189) -> ()
                    n170 = case shown="True" w183 {
                      tunnel: w187 -> [_ w205]
                      tunnel: w186 -> [_ w204]
                      frame #0 {
                      }
                      frame #1 {
                        n171 = stacked-sequence {
                          tunnel: w205 -> [w207 w229]
                          tunnel: w204 -> [w206 _]
                          frame #0 {
                            n172 = stacked-sequence {
                              tunnel: w207 -> [_ _ w218]
                              frame #0 {
                                w208 = 2
                                # "third axis"
                                n173 = property on="Current Position (µm)" class="Cluster (strict)"() -> ("Value"=w211:cluster{"x":dbl, "y":dbl, "z":dbl})  [unwired: 2 in, 2 out]
                                n174 = Cluster To Array(cluster=w211) -> (array=w209:dbl[])
                                n175 = Index Array(array=w209, index=w208) -> (element=w210:dbl)
                                n176 = call "SetAxisPos.vi"("Position"=w210, "Axis"=w208) -> ("error out"=w212:errorcluster)
                                n177 = call "HandleError.vi"("error in (no error)"=w212) -> ()
                              }
                              frame #1 {
                                n178 = call "HaltStageOutput.vi"() -> ("Error out"=w213:errorcluster)  [unwired: 1 in]
                                n179 = call "HandleError.vi"("error in (no error)"=w213) -> ()
                              }
                              frame #2 {
                                n180 = call "FIFOStopDAQ.vi"() -> ("error out"=w219:errorcluster)
                                n181 = call "StageType.vi"("Function"=T4."Get Type") -> ("Stage Type (output)"=w214:T9)  [unwired: 2 in, 2 out]
                                n182 = call "HandleError.vi"("error in (no error)"=w219) -> ()
                                n183 = case shown="\"PI analogue step\", Default" w214 {
                                tunnel: [w222 w223] -> w220
                                tunnel: enum16{"start", "state", "abort"}."abort" ("operation") -> [w221 w224]
                                frame #0 {
                                n184 = call "OperateOnAnalogOutput.vi"("operation"=w221) -> ("error out"=w222:errorcluster)  [unwired: 1 in, 1 out]
                                }
                                frame #1 {
                                n185 = call "OperateOnDigitalOutput.vi"("operation"=w224) -> ("error out"=w223:errorcluster)  [unwired: 3 in]
                                }
                                }
                                n186 = call "UpdateDAQLinescanDisplay.vi"("LinescanSampling"=w218, "operation"=enum16{"initialize", "update"}."update") -> ()  [unwired: 3 in]
                                n187 = call "HandleError.vi"("error in (no error)"=w220) -> ()
                              }
                            }
                            n188 = case shown="False" w206 {
                              frame #0 {
                              }
                              frame #1 {
                                n189 = call "FIFOFileObject.vi"(".sm file format"=FALSE, "function (open:0)"=enum16{"open", "write", "close"}."close") -> ("error out"=w226:errorcluster)  [unwired: 4 in]
                                n190 = call "HandleError.vi"("error in (no error)"=w226) -> ()
                              }
                            }
                          }
                          frame #1 {
                            n191 = local read "Image Settings"() -> (w231:T2)
                            n192 = call "NextLine.vi"("Image Settings"=w231) -> ("Continue Scan"=w228:bool)
                            n193 = case shown="True" w228 {
                              tunnel: w229 -> [w232 _]
                              frame #0 {
                                n194 = stacked-sequence {
                                tunnel: w232 -> [w233 _ _ _]
                                frame #0 {
                                n195 = call "ScannedImage.vi"("Get/Set"=TRUE, "Scanned Image (input)"=w233) -> ()  [unwired: 1 out]
                                }
                                frame #1 {
                                n196 = local read "Display Settings"() -> (w235:T1)
                                n197 = call "UpdateFullImage.vi"("Display Settings"=w235) -> ()
                                }
                                frame #2 {
                                n198 = property on="Current Position (µm)" class="Cluster (strict)"() -> ("Value"=w237:cluster{"x":dbl, "y":dbl, "z":dbl})  [unwired: 2 in, 2 out]
                                n199 = call "SetPosition.vi"("Current Position (µm)"=w237) -> ("error out"=w236:errorcluster)
                                n200 = call "HandleError.vi"("error in (no error)"=w236) -> ()
                                }
                                frame #3 {
                                w238 = FALSE ("Laser 1")
                                n201 = call "AOTFSetPosition.vi"() -> ()  [unwired: 2 in]
                                n202 = property on="Laser 4" class="Boolesch (strikt)"("Value"=w238) -> ()  [unwired: 2 in, 2 out]
                                n203 = property on="Laser 1" class="Boolean (strict)"("Value"=w238) -> ()  [unwired: 2 in, 2 out]
                                n204 = property on="Laser 2" class="Boolean (strict)"("Value"=w238) -> ()  [unwired: 2 in, 2 out]
                                n205 = property on="Laser 3" class="Boolean (strict)"("Value"=w238) -> ()  [unwired: 2 in, 2 out]
                                }
                                }
                              }
                              frame #1 {
                                # "show position at end of line"
                                n206 = case shown="False" "show position (PI digital)" {
                                frame #0 {
                                }
                                frame #1 {
                                n207 = call "POS?.vi"("System no."=1, "All axes?"=TRUE) -> ("Position"=→"Position":dbl[])  [unwired: 16 in, 1 out]
                                }
                                }
                              }
                            }
                            n208 = call "UpdateFrontPanel.vi"("operation"=enum16{"set references", "update"}."update", "Scan"=w228) -> ()  [unwired: 8 in]
                            n209 = property on="Scan" class="Boolean (strict)"("Value"=w228) -> ()  [unwired: 2 in, 2 out]
                          }
                        }
                      }
                    }
                  }
                }
              }
            }
          }
          event #1 {
            n210 = event-data() -> ()  [unwired: 1 in, 1 out]
            n211 = Unbundle By Name("Current Position (µm)") -> ("x"=w244:dbl)
            n212 = Unbundle By Name("Position Increment (µm)") -> ("x"=w248:dbl)
            n213 = Subtract(x=w244, y=w248) -> (x-y=w245:dbl)
            n214 = Bundle By Name(cluster="Current Position (µm)", "x"=w245) -> (w243:cluster{"x":dbl, "y":dbl, "z":dbl})
            n215 = local read "Scan"() -> (w249:bool)
            n216 = case shown="True" w249 {
              tunnel: w243 -> [w251 w256]
              frame #0 {
                n217 = call "SetPosition.vi"("Current Position (µm)"=w251) -> ("error out"=w250:errorcluster)
                n218 = call "HandleError.vi"("error in (no error)"=w250) -> ()
              }
              frame #1 {
                n219 = Cluster To Array(cluster=w256) -> (array=w255:dbl[])
                n220 = local read "Image Settings"() -> (w259:T2)
                n221 = Unbundle By Name(w259) -> ("1st Axis"=w258:u16, "2nd Axis"=w257:u16)
                n222 = call "GetThirdAxis.vi"("1st Axis"=w257, "2nd Axis"=w258) -> ("3rd Axis"=w254:i32)  [unwired: 2 in]
                n223 = Index Array(array=w255, index=w254) -> (element=w253:dbl)
                n224 = call "SetAxisPos.vi"("Position"=w253, "Axis"=w254) -> ("error out"=w252:errorcluster)
                n225 = call "HandleError.vi"("error in (no error)"=w252) -> ()
              }
            }
            n226 = local write "Current Position (µm)"(w243) -> ()
          }
          event #2 {
            n227 = event-data() -> ()  [unwired: 1 in, 1 out]
            n228 = local read "Position Increment (µm)"() -> (w263:cluster{"x":dbl, "y":dbl, "z":dbl})
            n229 = local read "Current Position (µm)"() -> (w264:cluster{"x":dbl, "y":dbl, "z":dbl})
            n230 = Unbundle By Name(w264) -> ("x"=w265:dbl)
            n231 = Unbundle By Name(w263) -> ("x"=w262:dbl)
            n232 = Add(x=w265, y=w262) -> (x+y=w266:dbl)
            n233 = local read "Scan"() -> (w261:bool)
            n234 = Bundle By Name(cluster=w264, "x"=w266) -> (w260:cluster{"x":dbl, "y":dbl, "z":dbl})
            n235 = local write "Current Position (µm)"(w260) -> ()
            n236 = case shown="False" w261 {
              tunnel: w260 -> [w268 w271]
              frame #0 {
                n237 = call "SetPosition.vi"("Current Position (µm)"=w268) -> ("error out"=w267:errorcluster)
                n238 = call "HandleError.vi"("error in (no error)"=w267) -> ()
              }
              frame #1 {
                n239 = Cluster To Array(cluster=w271) -> (array=w273:dbl[])
                n240 = local read "Image Settings"() -> (w276:T2)
                n241 = Unbundle By Name(w276) -> ("1st Axis"=w275:u16, "2nd Axis"=w274:u16)
                n242 = call "GetThirdAxis.vi"("1st Axis"=w274, "2nd Axis"=w275) -> ("3rd Axis"=w272:i32)  [unwired: 2 in]
                n243 = Index Array(array=w273, index=w272) -> (element=w270:dbl)
                n244 = call "SetAxisPos.vi"("Position"=w270, "Axis"=w272) -> ("error out"=w269:errorcluster)
                n245 = call "HandleError.vi"("error in (no error)"=w269) -> ()
              }
            }
          }
          event #3 {
            n246 = event-data() -> ()  [unwired: 1 in, 1 out]
            n247 = local read "Position Increment (µm)"() -> (w282:cluster{"x":dbl, "y":dbl, "z":dbl})
            n248 = local read "Current Position (µm)"() -> (w279:cluster{"x":dbl, "y":dbl, "z":dbl})
            n249 = Unbundle By Name(w279) -> ("y"=w281:dbl)
            n250 = Unbundle By Name(w282) -> ("y"=w280:dbl)
            n251 = Add(x=w281, y=w280) -> (x+y=w283:dbl)
            n252 = local read "Scan"() -> (w278:bool)
            n253 = Bundle By Name(cluster=w279, "y"=w283) -> (w277:cluster{"x":dbl, "y":dbl, "z":dbl})
            n254 = local write "Current Position (µm)"(w277) -> ()
            n255 = case shown="False" w278 {
              tunnel: w277 -> [w285 w288]
              frame #0 {
                n256 = call "SetPosition.vi"("Current Position (µm)"=w285) -> ("error out"=w284:errorcluster)
                n257 = call "HandleError.vi"("error in (no error)"=w284) -> ()
              }
              frame #1 {
                n258 = Cluster To Array(cluster=w288) -> (array=w290:dbl[])
                n259 = local read "Image Settings"() -> (w293:T2)
                n260 = Unbundle By Name(w293) -> ("1st Axis"=w292:u16, "2nd Axis"=w291:u16)
                n261 = call "GetThirdAxis.vi"("1st Axis"=w291, "2nd Axis"=w292) -> ("3rd Axis"=w289:i32)  [unwired: 2 in]
                n262 = Index Array(array=w290, index=w289) -> (element=w287:dbl)
                n263 = call "SetAxisPos.vi"("Position"=w287, "Axis"=w289) -> ("error out"=w286:errorcluster)
                n264 = call "HandleError.vi"("error in (no error)"=w286) -> ()
              }
            }
          }
          event #4 {
            n265 = event-data() -> ()  [unwired: 1 in, 1 out]
            n266 = local read "Position Increment (µm)"() -> (w298:cluster{"x":dbl, "y":dbl, "z":dbl})
            n267 = local read "Current Position (µm)"() -> (w299:cluster{"x":dbl, "y":dbl, "z":dbl})
            n268 = Unbundle By Name(w299) -> ("y"=w296:dbl)
            n269 = Unbundle By Name(w298) -> ("y"=w297:dbl)
            n270 = Subtract(x=w296, y=w297) -> (x-y=w300:dbl)
            n271 = Bundle By Name(cluster=w299, "y"=w300) -> (w294:cluster{"x":dbl, "y":dbl, "z":dbl})
            n272 = local read "Scan"() -> (w295:bool)
            n273 = local write "Current Position (µm)"(w294) -> ()
            n274 = case shown="False" w295 {
              tunnel: w294 -> [w302 w305]
              frame #0 {
                n275 = call "SetPosition.vi"("Current Position (µm)"=w302) -> ("error out"=w301:errorcluster)
                n276 = call "HandleError.vi"("error in (no error)"=w301) -> ()
              }
              frame #1 {
                n277 = Cluster To Array(cluster=w305) -> (array=w307:dbl[])
                n278 = local read "Image Settings"() -> (w310:T2)
                n279 = Unbundle By Name(w310) -> ("1st Axis"=w309:u16, "2nd Axis"=w308:u16)
                n280 = call "GetThirdAxis.vi"("1st Axis"=w308, "2nd Axis"=w309) -> ("3rd Axis"=w306:i32)  [unwired: 2 in]
                n281 = Index Array(array=w307, index=w306) -> (element=w304:dbl)
                n282 = call "SetAxisPos.vi"("Position"=w304, "Axis"=w306) -> ("error out"=w303:errorcluster)
                n283 = call "HandleError.vi"("error in (no error)"=w303) -> ()
              }
            }
          }
          event #5 {
            n284 = event-data() -> ()  [unwired: 1 in, 1 out]
            n285 = local read "Position Increment (µm)"() -> (w316:cluster{"x":dbl, "y":dbl, "z":dbl})
            n286 = local read "Current Position (µm)"() -> (w313:cluster{"x":dbl, "y":dbl, "z":dbl})
            n287 = Unbundle By Name(w316) -> ("z"=w314:dbl)
            n288 = Unbundle By Name(w313) -> ("z"=w315:dbl)
            n289 = Add(x=w315, y=w314) -> (x+y=w317:dbl)
            n290 = Bundle By Name(cluster=w313, "z"=w317) -> (w311:cluster{"x":dbl, "y":dbl, "z":dbl})
            n291 = local write "Current Position (µm)"(w311) -> ()
            n292 = local read "Scan"() -> (w312:bool)
            n293 = case shown="False" w312 {
              tunnel: w311 -> [w319 w322]
              frame #0 {
                n294 = call "SetPosition.vi"("Current Position (µm)"=w319) -> ("error out"=w318:errorcluster)
                n295 = call "HandleError.vi"("error in (no error)"=w318) -> ()
              }
              frame #1 {
                n296 = Cluster To Array(cluster=w322) -> (array=w324:dbl[])
                n297 = local read "Image Settings"() -> (w327:T2)
                n298 = Unbundle By Name(w327) -> ("1st Axis"=w326:u16, "2nd Axis"=w325:u16)
                n299 = call "GetThirdAxis.vi"("1st Axis"=w325, "2nd Axis"=w326) -> ("3rd Axis"=w323:i32)  [unwired: 2 in]
                n300 = Index Array(array=w324, index=w323) -> (element=w321:dbl)
                n301 = call "SetAxisPos.vi"("Position"=w321, "Axis"=w323) -> ("error out"=w320:errorcluster)
                n302 = call "HandleError.vi"("error in (no error)"=w320) -> ()
              }
            }
          }
          event #6 {
            n303 = event-data() -> ()  [unwired: 1 in, 1 out]
            n304 = local read "Position Increment (µm)"() -> (w334:cluster{"x":dbl, "y":dbl, "z":dbl})
            n305 = local read "Current Position (µm)"() -> (w330:cluster{"x":dbl, "y":dbl, "z":dbl})
            n306 = Unbundle By Name(w330) -> ("z"=w333:dbl)
            n307 = Unbundle By Name(w334) -> ("z"=w332:dbl)
            n308 = Subtract(x=w333, y=w332) -> (x-y=w331:dbl)
            n309 = Bundle By Name(cluster=w330, "z"=w331) -> (w328:cluster{"x":dbl, "y":dbl, "z":dbl})
            n310 = local read "Scan"() -> (w329:bool)
            n311 = local write "Current Position (µm)"(w328) -> ()
            n312 = case shown="False" w329 {
              tunnel: w328 -> [w336 w339]
              frame #0 {
                n313 = call "SetPosition.vi"("Current Position (µm)"=w336) -> ("error out"=w335:errorcluster)
                n314 = call "HandleError.vi"("error in (no error)"=w335) -> ()
              }
              frame #1 {
                n315 = Cluster To Array(cluster=w339) -> (array=w341:dbl[])
                n316 = local read "Image Settings"() -> (w344:T2)
                n317 = Unbundle By Name(w344) -> ("1st Axis"=w343:u16, "2nd Axis"=w342:u16)
                n318 = call "GetThirdAxis.vi"("1st Axis"=w342, "2nd Axis"=w343) -> ("3rd Axis"=w340:i32)  [unwired: 2 in]
                n319 = Index Array(array=w341, index=w340) -> (element=w338:dbl)
                n320 = call "SetAxisPos.vi"("Position"=w338, "Axis"=w340) -> ("error out"=w337:errorcluster)
                n321 = call "HandleError.vi"("error in (no error)"=w337) -> ()
              }
            }
          }
          event #7 {
            n322 = event-data() -> ()  [unwired: 1 in, 1 out]
            n323 = local read "Current Position (µm)"() -> (w345:cluster{"x":dbl, "y":dbl, "z":dbl})
            n324 = Unbundle By Name(w345) -> ("x"=w351:dbl, "y"=w350:dbl, "z"=w348:dbl)
            n325 = Bundle("x"=w351, "y"=w350, "z"=w348) -> (w349:cluster{"x":dbl, "y":dbl, "z":dbl})  [unwired: 1 in]
            n326 = case shown="False" "Keep Start Position" {
              tunnel: w349 -> [w352 w362]
              tunnel: "Keep Image Size" -> [w353 w363]
              frame #0 {
                n327 = property on="Start Position (µm)" class="Clust (strict)"("Value"=w352) -> ()  [unwired: 2 in, 2 out]
                n328 = case shown="False" w353 {
                  tunnel: w352 -> [w354 w357]
                  frame #0 {
                    n329 = property on="Image Size (µm)" class="Clust (strict)"() -> ("Value"=w355:cluster{"x":dbl, "y":dbl, "z":dbl})  [unwired: 2 in, 2 out]
                    n330 = Add(x=w355, y=w354) -> (x+y=w356:cluster{"x":dbl, "y":dbl, "z":dbl})
                    n331 = property on="End Position (µm)" class="Clust (strict)"("Value"=w356) -> ()  [unwired: 2 in, 2 out]
                  }
                  frame #1 {
                    n332 = stacked-sequence {
                      tunnel: w357 -> [w358 _]
                      frame #0 {
                        n333 = property on="End Position (µm)" class="Clust (strict)"() -> ("Value"=w360:cluster{"x":dbl, "y":dbl, "z":dbl})  [unwired: 2 in, 2 out]
                        n334 = Subtract(x=w360, y=w358) -> (x-y=w359:cluster{"x":dbl, "y":dbl, "z":dbl})
                        n335 = property on="Image Size (µm)" class="Clust (strict)"("Value"=w359) -> ()  [unwired: 2 in, 2 out]
                      }
                      frame #1 {
                        n336 = call "UpdateImageInfo.vi"("operation"=enum16{"set references", "update"}."update") -> ()  [unwired: 3 in]
                      }
                    }
                  }
                }
              }
              frame #1 {
                n337 = property on="End Position (µm)" class="Clust (strict)"("Value"=w362) -> ()  [unwired: 2 in, 2 out]
                n338 = case shown="False" w363 {
                  tunnel: w362 -> [w364 w367]
                  frame #0 {
                    n339 = property on="Image Size (µm)" class="Clust (strict)"() -> ("Value"=w366:cluster{"x":dbl, "y":dbl, "z":dbl})  [unwired: 2 in, 2 out]
                    n340 = Subtract(x=w364, y=w366) -> (x-y=w365:cluster{"x":dbl, "y":dbl, "z":dbl})
                    n341 = property on="Start Position (µm)" class="Clust (strict)"("Value"=w365) -> ()  [unwired: 2 in, 2 out]
                  }
                  frame #1 {
                    n342 = stacked-sequence {
                      tunnel: w367 -> [w368 _]
                      frame #0 {
                        n343 = property on="Start Position (µm)" class="Clust (strict)"() -> ("Value"=w370:cluster{"x":dbl, "y":dbl, "z":dbl})  [unwired: 2 in, 2 out]
                        n344 = Subtract(x=w368, y=w370) -> (x-y=w369:cluster{"x":dbl, "y":dbl, "z":dbl})
                        n345 = property on="Image Size (µm)" class="Clust (strict)"("Value"=w369) -> ()  [unwired: 2 in, 2 out]
                      }
                      frame #1 {
                        n346 = call "UpdateImageInfo.vi"("operation"=enum16{"set references", "update"}."update") -> ()  [unwired: 3 in]
                      }
                    }
                  }
                }
              }
            }
          }
          event #8 {
            n347 = event-data() -> ("NewVal"=w373:bool)  [unwired: 1 in]
            n348 = control-ref of="y"() -> (w374:refnum<vi>)
            n349 = case shown="True" w373 {
              frame #0 {
              }
              frame #1 {
                n350 = stacked-sequence {
                  frame #0 {
                    n351 = property on="Image Resolution (nm/pixel)" class="Clust (strict)"() -> ("Value"=w378:cluster{"x":dbl, "y":dbl, "z":dbl})  [unwired: 2 in, 2 out]
                    n352 = Unbundle(w378) -> ("x"=w377:dbl, "z"=w375:dbl)  [unwired: 1 out]
                    n353 = Bundle("x"=w377, "x"=w377, "z"=w375) -> (w376:cluster{"x":dbl, "x":dbl, "z":dbl})  [unwired: 1 in]
                    n354 = property on="Image Resolution (nm/pixel)" class="Clust (strict)"("Value"=w376) -> ()  [unwired: 2 in, 2 out]
                  }
                  frame #1 {
                    n355 = call "UpdateImageInfo.vi"() -> ()  [unwired: 4 in]
                  }
                }
              }
            }
            n356 = Not(x=w373) -> (.not. x?=w372:bool)
            n357 = call "EnableControl.vi"("Enable"=w372, "Reference"=w374) -> ()
          }
          event #9 {
            n358 = event-data() -> ("NewVal"=w380:cluster{"x":dbl, "y":dbl, "z":dbl})  [unwired: 1 in]
            n359 = local read "Keep Image Size"() -> (w379:bool)
            n360 = case shown="False" w379 {
              tunnel: w380 -> [w383 w384]
              frame #0 {
                n361 = property on="Image Size (µm)" class="Clust (strict)"() -> ("Value"=w381:cluster{"x":dbl, "y":dbl, "z":dbl})  [unwired: 2 in, 2 out]
                n362 = Add(x=w381, y=w383) -> (x+y=w382:cluster{"x":dbl, "y":dbl, "z":dbl})
                n363 = property on="End Position (µm)" class="Clust (strict)"("Value"=w382) -> ()  [unwired: 2 in, 2 out]
              }
              frame #1 {
                n364 = stacked-sequence {
                  tunnel: w384 -> [w387 _]
                  frame #0 {
                    n365 = property on="End Position (µm)" class="Cluster (strict)"() -> ("Value"=w386:cluster{"x":dbl, "y":dbl, "z":dbl})  [unwired: 2 in, 2 out]
                    n366 = Subtract(x=w386, y=w387) -> (x-y=w385:cluster{"x":dbl, "y":dbl, "z":dbl})
                    n367 = property on="Image Size (µm)" class="Cluster (strict)"("Value"=w385) -> ()  [unwired: 2 in, 2 out]
                  }
                  frame #1 {
                    n368 = call "UpdateImageInfo.vi"() -> ()  [unwired: 4 in]
                  }
                }
              }
            }
          }
          event #10 {
            n369 = event-data() -> ("NewVal"=w389:cluster{"x":dbl, "y":dbl, "z":dbl})  [unwired: 1 in]
            n370 = local read "Keep Image Size"() -> (w388:bool)
            n371 = case shown="False" w388 {
              tunnel: w389 -> [w391 w393]
              frame #0 {
                n372 = property on="Image Size (µm)" class="Clust (strict)"() -> ("Value"=w392:cluster{"x":dbl, "y":dbl, "z":dbl})  [unwired: 2 in, 2 out]
                n373 = Subtract(x=w391, y=w392) -> (x-y=w390:cluster{"x":dbl, "y":dbl, "z":dbl})
                n374 = property on="Start Position (µm)" class="Clust (strict)"("Value"=w390) -> ()  [unwired: 2 in, 2 out]
              }
              frame #1 {
                n375 = stacked-sequence {
                  tunnel: w393 -> [w396 _]
                  frame #0 {
                    n376 = property on="Start Position (µm)" class="Clust (strict)"() -> ("Value"=w395:cluster{"x":dbl, "y":dbl, "z":dbl})  [unwired: 2 in, 2 out]
                    n377 = Subtract(x=w396, y=w395) -> (x-y=w394:cluster{"x":dbl, "y":dbl, "z":dbl})
                    n378 = property on="Image Size (µm)" class="Clust (strict)"("Value"=w394) -> ()  [unwired: 2 in, 2 out]
                  }
                  frame #1 {
                    n379 = call "UpdateImageInfo.vi"() -> ()  [unwired: 4 in]
                  }
                }
              }
            }
          }
          event #11 {
            n380 = event-data() -> ("NewVal"=w397:cluster{"x":dbl, "y":dbl, "z":dbl})  [unwired: 1 in]
            n381 = stacked-sequence {
              tunnel: w397 -> [w399 _]
              frame #0 {
                n382 = local read "Keep Start Position"() -> (w398:bool)
                n383 = case shown="False" w398 {
                  tunnel: w399 -> [w400 w403]
                  frame #0 {
                    n384 = property on="Start Position (µm)" class="Clust (strict)"() -> ("Value"=w402:cluster{"x":dbl, "y":dbl, "z":dbl})  [unwired: 2 in, 2 out]
                    n385 = Add(x=w400, y=w402) -> (x+y=w401:cluster{"x":dbl, "y":dbl, "z":dbl})
                    n386 = property on="End Position (µm)" class="Clust (strict)"("Value"=w401) -> ()  [unwired: 2 in, 2 out]
                  }
                  frame #1 {
                    n387 = property on="End Position (µm)" class="Clust (strict)"() -> ("Value"=w404:cluster{"x":dbl, "y":dbl, "z":dbl})  [unwired: 2 in, 2 out]
                    n388 = Subtract(x=w404, y=w403) -> (x-y=w405:cluster{"x":dbl, "y":dbl, "z":dbl})
                    n389 = property on="Start Position (µm)" class="Clust (strict)"("Value"=w405) -> ()  [unwired: 2 in, 2 out]
                  }
                }
              }
              frame #1 {
                n390 = call "UpdateImageInfo.vi"("operation"=enum16{"set references", "update"}."update") -> ()  [unwired: 3 in]
              }
            }
          }
          event #12 {
            n391 = event-data() -> ()  [unwired: 1 in, 5 out]
            n392 = call "UpdateImageInfo.vi"() -> ()  [unwired: 4 in]
            n393 = local read "Image Settings"() -> (w415:T2)
            n394 = Unbundle By Name(w415) -> ("Time Resolution\n(ms/pixel)"=w414:dbl)
            n395 = Reciprocal(x=w414) -> (1/x=w413:dbl)
            n396 = Select(t=w413, s="x-scale: Time?", f=1.0) -> (s? t:f=w412:dbl)
            n397 = Select(t="Time [ms]", s="x-scale: Time?", f="Pixel") -> (s? t:f=w409:string)
            n398 = property on="MCS Trace" class="WaveformChart (strict)"("X Scale.Offset and Multiplier:Multiplier"=w412, "X Scale.Name Label.Text"=w409) -> ()  [unwired: 2 in, 2 out]
          }
          event #13 {
            n399 = event-data() -> ("NewVal"=w420:bool)  [unwired: 1 in, 4 out]
            n400 = property on="Show Image" class="Boolean (strict)"() -> ("Value"=w416:bool)  [unwired: 2 in, 2 out]
            n401 = call "DAQLinescanVisualization.vi"() -> ("Visualization (output)"=w419:T6)  [unwired: 2 in]
            n402 = And(x=w420, y=w416) -> (x .and. y?=w417:bool)
            n403 = Unbundle By Name(w419) -> ("Retrace Window #"=w418:u32)
            n404 = call "IMAQ WindShow"("Bring To Front? (N)"=w417, "Hide/Show (Show)"=w417, "Window Number (0...15)"=w418) -> ()  [unwired: 3 in, 3 out]
          }
          event #14 {
            n405 = event-data() -> ("Time"=w421:u32, "NewVal"=w423:bool)  [unwired: 1 in, 3 out]
            n406 = call "DAQLinescanVisualization.vi"() -> ("Visualization (output)"=w429:T6)  [unwired: 2 in]
            n407 = property on="Retrace" class="Boolean (strict)"() -> ("Value"=w425:bool)  [unwired: 2 in, 2 out]
            n408 = Unbundle By Name(w429) -> ("Trace Window #"=w428:u32, "Retrace Window #"=w427:u32)
            n409 = control-ref of="Plane"() -> (w424:refnum<vi>)
            n410 = And(x=w425, y=w423) -> (x .and. y?=w426:bool)
            n411 = Multiply(x=w421, y=w428) -> (x*y=w422:u32)
            n412 = call "IMAQ WindToolsShow"("Hide/Show (Show)"=w423) -> ()  [unwired: 4 in, 2 out]
            n413 = call "IMAQ WindShow"("Bring To Front? (N)"=w423, "Hide/Show (Show)"=w423, "Window Number (0...15)"=w422) -> ()  [unwired: 3 in, 3 out]
            n414 = call "IMAQ WindShow"("Bring To Front? (N)"=w426, "Hide/Show (Show)"=w426, "Window Number (0...15)"=w427) -> ()  [unwired: 3 in, 3 out]
            n415 = call "EnableControl.vi"("Enable"=w423, "Reference"=w424) -> ()
          }
          event #15 {
            n416 = event-data() -> ()  [unwired: 1 in, 5 out]
            n417 = control-ref of="Load Image"() -> (w430:refnum<vi>)
            n418 = control-ref of="Scan"() -> ()  [unwired: 1 out]
            n419 = call "BuildHdrFilePath.vi"("Destination:"="Destination:") -> ("error in (no error)"=w432:errorcluster, "configuration file path"=w433:path)  [unwired: 1 in]
            n420 = call "UpdateSomeButtons.vi"("Load"=w430, "Destination:"=w433, "error in (no error)"=w432, "Store Data"="Store Data") -> ("error"=w431:errorcluster)  [unwired: 1 in]
            n421 = call "HandleError.vi"("error in (no error)"=w431) -> ()
          }
          event #16 {
            n422 = event-data() -> ()  [unwired: 1 in, 5 out]
            n423 = Select(t=u8 2 ("Y Scale.Scale Fit"), s="Autoscale y-axis", f=u8 0 ("Y Scale.Scale Fit")) -> (s? t:f=w438:u8)
            n424 = property on="MCS Trace" class="WaveformChart (strict)"("Y Scale.Scale Fit"=w438) -> ()  [unwired: 2 in, 2 out]
          }
          event #17 {
            n425 = event-data() -> ()  [unwired: 1 in, 5 out]
            n426 = property on="Scan" class="Boolean (strict)"() -> ("Value"=w440:bool)  [unwired: 2 in, 2 out]
            n427 = case shown="False" w440 {
              frame #0 {
                n428 = call "UpdateFullImage.vi"("Display Settings"="Display Settings") -> ()
              }
              frame #1 {
              }
            }
          }
          event #18 {
            n429 = event-data() -> ()  [unwired: 1 in, 1 out]
            n430 = case shown="True" "EOM Setup" {
              frame #0 {
              }
              frame #1 {
                n431 = stacked-sequence {
                  frame #0 {
                    n432 = property class="VI"() -> ("VI Name"=w444:string)  [unwired: 2 in, 2 out]
                    n433 = call "CallersName.vi"("Get/Set"=TRUE ("s"), "Callers Name"=w444) -> ()  [unwired: 1 out]
                  }
                  frame #1 {
                    n434 = call "SetupEOM.vi"() -> ()  [unwired: 1 in]
                  }
                }
              }
            }
          }
          event #19 {
            n435 = event-data() -> ("NewVal"=w446:u16)  [unwired: 1 in, 4 out]
            n436 = flat-sequence {
              tunnel: w446 -> [w451]
              tunnel: [w451] -> w445
              tunnel: w445 -> [w455]
              frame #0 {
                n437 = property on="AOTF" class="Ring (strict)"() -> ("Value"=w448:u16)  [unwired: 2 in, 2 out]
                n438 = Not Equal To 0?(x=w451) -> (x != 0?=w452:bool)
                n439 = Equal?(x=u8 7, y=w448) -> (x = y?=w447:bool)
                n440 = And(x=w452, y=w447) -> (x .and. y?=w450:bool)
                n441 = case shown="True" w450 {
                  frame #0 {
                  }
                  frame #1 {
                    w454 = u16 3 items=["None", "Laser 1", "Laser 2", "Laser 1 + 2", "Laser 3", "Laser 1 + 3", "Laser 2 + 3", "Laser 1+2+3"] ("AOTF")
                    n442 = control-ref of="AOTF"() -> (w453:refnum<vi>)
                    n443 = call "Display Message to User"() -> ()  [unwired: 10 in, 2 out]
                    n444 = property on="Property Node" class="Ring (strict)"(reference=w453, "Value"=w454) -> ()  [unwired: 1 in, 2 out]
                  }
                }
              }
              frame #1 {
                n445 = case shown="1, Default" w455 {
                  frame #0 {
                  }
                  frame #1 {
                    n446 = call "EOMSetPosition.vi"("value"=sgl 0.0) -> ()
                  }
                }
              }
            }
          }
          event #20 {
            n447 = event-data() -> ()  [unwired: 1 in, 1 out]
            n448 = case shown="True" "Stage Setup" {
              frame #0 {
              }
              frame #1 {
                n449 = stacked-sequence {
                  frame #0 {
                    n450 = call "StageType.vi"() -> ()  [unwired: 3 in, 3 out]
                  }
                  frame #1 {
                    n451 = call "SetupStage.vi"() -> ()  [unwired: 1 in]
                  }
                  frame #2 {
                    n452 = call "StageInit.vi"() -> ("error out"=w458:errorcluster)  [unwired: 1 in]
                    n453 = case shown="No Error" w458 {
                      selector: w458 -> [_ w462]
                      tunnel: [w460 w462] -> w459
                      frame #0 {
                        n454 = property on="Current Position (µm)" class="Clust (strict)"() -> ("Value"=w461:cluster{"x":dbl, "y":dbl, "z":dbl})  [unwired: 2 in, 2 out]
                        n455 = call "SetPosition.vi"("Current Position (µm)"=w461) -> ("error out"=w460:errorcluster)
                      }
                      frame #1 {
                      }
                    }
                    n456 = call "HandleError.vi"("error in (no error)"=w459) -> ()
                  }
                }
              }
            }
          }
          event #21 {
            n457 = event-data() -> ()  [unwired: 1 in, 6 out]
            n458 = case shown="True" "AOTF Setup" {
              frame #0 {
              }
              frame #1 {
                n459 = stacked-sequence {
                  frame #0 {
                    n460 = property class="VI"() -> ("VI Name"=w465:string)  [unwired: 2 in, 2 out]
                    n461 = call "CallersName.vi"("Get/Set"=TRUE ("s"), "Callers Name"=w465) -> ()  [unwired: 1 out]
                  }
                  frame #1 {
                    n462 = call "SetupAOTF.vi"() -> ()  [unwired: 1 in]
                  }
                }
              }
            }
          }
          event #22 {
            n463 = event-data() -> ("NewVal"=w466:u16)  [unwired: 1 in, 5 out]
            n464 = flat-sequence {
              tunnel: w466 -> [w467]
              frame #0 {
                n465 = Equal?(x=u8 7, y=w467) -> (x = y?=w472:bool)
                n466 = property on="EOM" class="Ring (strict)"() -> ("Value"=w468:u16)  [unwired: 2 in, 2 out]
                n467 = Not Equal To 0?(x=w468) -> (x != 0?=w469:bool)
                n468 = And(x=w469, y=w472) -> (x .and. y?=w470:bool)
                n469 = case shown="True" w470 {
                  frame #0 {
                  }
                  frame #1 {
                    w473 = u16 3 items=["None", "Laser 1", "Laser 2", "Laser 1 + 2", "Laser 3", "Laser 1 + 3", "Laser 2 + 3", "Laser 1+2+3"] ("AOTF")
                    n470 = call "Display Message to User2"() -> ()  [unwired: 10 in, 2 out]
                    n471 = property on="AOTF" class="Ring (strict)"("Value"=w473) -> ()  [unwired: 2 in, 2 out]
                  }
                }
              }
              frame #1 {
                n472 = call "AOTFSetPosition.vi"() -> ()  [unwired: 2 in]
              }
            }
          }
          event #23 {
            n473 = event-data() -> ("ItemTag"=w474:string)  [unwired: 1 in, 5 out]
            n474 = case shown="\"\", Default" w474 {
              frame #0 {
              }
              frame #1 {
                n475 = call "Splashscreen.vi"("Mode"=enum16{"splash", "dialog"}."dialog") -> ()  [unwired: 1 in]
              }
            }
          }
          event #24 {
            n476 = event-data() -> ()  [unwired: 1 in, 1 out]
            n477 = case shown="True" "SPC Setup" {
              frame #0 {
              }
              frame #1 {
                n478 = stacked-sequence {
                  frame #0 {
                    w477 = u16 1 items=["standalone", "dialog"] ("mode")
                    n479 = call "DAQFIFO_HH.vi"("mode"=w477) -> ()
                  }
                  frame #1 {
                    n480 = call "FIFOSettings.vi"() -> ("FIFO Settings(out)"=w478:T5)  [unwired: 2 in]
                    n481 = call "SPCSetParameters_HH.vi"("FIFO Settings"=w478) -> ("error (out)"=w479:errorcluster)  [unwired: 2 in]
                    n482 = call "HandleError.vi"("error in (no error)"=w479) -> ()
                  }
                  frame #2 {
                    n483 = property class="VI"() -> (error out=w480:errorcluster, "Front Panel"=w481:refnum<vi>)  [unwired: 2 in, 1 out]
                    n484 = call "UpdateDAQLinescanStatus.vi"("error in (no error)"=w480, "Panel"=w481) -> ()
                  }
                }
              }
            }
          }
          event #25 {
            n485 = event-data() -> ()  [unwired: 1 in, 1 out]
            n486 = stacked-sequence {
              frame #0 {
                n487 = case shown="True" "Save & Exit" {
                  frame #0 {
                  }
                  frame #1 {
                    n488 = call "WriteAnalogSettings.vi"() -> ("error out"=w487:errorcluster)  [unwired: 1 in]
                    n489 = call "WriteStageSettings.vi"("error in (no error)"=w487) -> ("error out"=w486:errorcluster)
                    n490 = call "WriteEOMSettings.vi"("error in (no error)"=w486) -> ("error out"=w485:errorcluster)
                    n491 = call "WriteAOTFSettings.vi"("error in (no error)"=w485) -> ("error out"=w484:errorcluster)
                    n492 = call "HandleError.vi"("error in (no error)"=w484) -> ()
                  }
                }
              }
              frame #1 {
                n493 = property class="VI"("Front Panel Window:Open"=TRUE) -> ()  [unwired: 2 in, 2 out]
              }
            }
          }
          event #26 {
            n494 = event-data() -> ("NewVal"=w489:bool)  [unwired: 1 in]
            n495 = call "UpdateFrontPanel.vi"("operation"=enum16{"set references", "update"}."update", "Scan"=w489) -> ()  [unwired: 8 in]
            n496 = case shown="True" w489 {
              frame #0 {
                n497 = stacked-sequence {
                  frame #0 {
                    n498 = call "OperateOnAnalogOutput.vi"("operation"=enum16{"start", "state", "abort"}."abort") -> ("error out"=w491:errorcluster)  [unwired: 1 in, 1 out]
                    n499 = call "HandleError.vi"("error in (no error)"=w491) -> ()
                  }
                  frame #1 {
                    n500 = call "HaltStageOutput.vi"() -> ("Error out"=w493:errorcluster)  [unwired: 1 in]
                    n501 = call "HandleError.vi"("error in (no error)"=w493) -> ()
                  }
                  frame #2 {
                    n502 = call "FIFOStopDAQ.vi"() -> ("error out"=w494:errorcluster)
                    n503 = call "HandleError.vi"("error in (no error)"=w494) -> ()
                  }
                  frame #3 {
                    n504 = property on="Current Position (µm)" class="Cluster (strict)"() -> ("Value"=w496:cluster{"x":dbl, "y":dbl, "z":dbl})  [unwired: 2 in, 2 out]
                    n505 = call "SetPosition.vi"("Current Position (µm)"=w496) -> ("error out"=w495:errorcluster)
                    n506 = call "HandleError.vi"("error in (no error)"=w495) -> ()
                  }
                  frame #4 {
                    n507 = call "FIFOFileObject.vi"(".sm file format"=FALSE, "function (open:0)"=enum16{"open", "write", "close"}."close") -> ("error out"=w499:errorcluster)  [unwired: 4 in]
                    n508 = call "HandleError.vi"("error in (no error)"=w499) -> ()
                  }
                  frame #5 {
                    n509 = call "UpdateDAQLinescanImage.vi"("operation"=enum16{"initialize", "update", "read"}."read") -> ("LinescanSampling"=w502:T11)  [unwired: 3 in, 1 out]
                    n510 = call "ScannedImage.vi"("Get/Set"=TRUE, "Scanned Image (input)"=w502) -> ()  [unwired: 1 out]
                  }
                  frame #6 {
                    n511 = local read "Display Settings"() -> (w503:T1)
                    n512 = call "UpdateFullImage.vi"("Display Settings"=w503) -> ()
                  }
                  frame #7 {
                    n513 = call "AOTFSetPosition.vi"() -> ()  [unwired: 2 in]
                  }
                }
              }
              frame #1 {
                n514 = call <vilib>:"Initialize Mouse.vi"() -> ("device ID"=w508:refnum<k1>)  [unwired: 10 in, 1 out]
                n515 = call-poly <vilib>:"Acquire Input Data.vi"("device ID"=w508) -> ("device ID"=w506:refnum<k1>, "axis info"=w507:T12)  [unwired: 15 in, 2 out]
                n516 = Unbundle By Name(w507) -> ("Scrolling"=w505:i32)
                n517 = Bundle("device ID"=w506, "Scrolling"=w505) -> (→"mouse focus":cluster{"device ID":refnum<k1>, "Scrolling":i32})  [unwired: 1 in]
                n518 = call "InitializeAnalogOutput.vi"("AOTF"="AOTF", "% puls-duration"=100.0, "Image Settings"="Image Settings", "EOM"="EOM") -> ("Error out"=w513:errorcluster)
                n519 = case shown="No Error" w513 {
                  selector: w513 -> [w516 w542]
                  tunnel: "Image Settings" -> [w518 _]
                  tunnel: [w517 w542] -> w512
                  frame #0 {
                    w536 = u16 0 items=["initialize", "update"] ("operation")
                    n520 = Unbundle By Name(w518) -> ("1st Axis"=w528:u16, "2nd Axis"=w529:u16, "Image Size (pixel)"=w530:cluster{"x":u32, "y":u32, "z":u32})
                    n521 = control-ref of="MCS Trace"() -> (w533:refnum<vi>)
                    n522 = call "FIFOInitDAQ_HH.vi"() -> ()  [unwired: 1 in]
                    n523 = control-ref of="Image Settings"() -> (w534:refnum<vi>)
                    n524 = control-ref of="Display Settings"() -> (w535:refnum<vi>)
                    n525 = Cluster To Array(cluster=w530) -> (array=w527:u32[])
                    n526 = call "GetThirdAxis.vi"("1st Axis"=w529, "2nd Axis"=w528) -> ("3rd Axis"=w526:i32)  [unwired: 2 in]
                    n527 = call "UpdateDAQLinescanDisplay.vi"("MCS Trace"=w533, "operation"=enum16{"initialize", "update"}."initialize", "Display Settings"=w535, "Image Settings"=w534) -> ()  [unwired: 1 in]
                    n528 = Index Array(array=w527, index=w526) -> (element=w524:u32)
                    n529 = call "ImageParameters.vi"("Get/Set"=TRUE, "Image Parameters (input)"=w518) -> ()  [unwired: 1 out]
                    n530 = property on="Store Data" class="Boolean (strict)"() -> ("Value"=w519:bool)  [unwired: 2 in, 2 out]
                    n531 = call "UpdateDAQLinescanImage.vi"("Image Settings"=w534, "operation"=w536) -> ()  [unwired: 2 in, 2 out]
                    n532 = Not Equal To 0?(x=w524) -> (x != 0?=w525:bool)
                    n533 = Decrement(x=w524) -> (x-1=w520:u32)
                    n534 = case shown="False" w519 {
                      tunnel: w518 -> [_ w540]
                      tunnel: [w537 w539] -> w517
                      tunnel: w516 -> [w537 w538]
                      frame #0 {
                      }
                      frame #1 {
                        n535 = property on="Destination:" class="Path"() -> ("Value"=w541:path)  [unwired: 2 in, 2 out]
                        n536 = call "WriteLinescanHeader.vi"("error in"=w538, "Destination:"=w541, "Image Settings"=w540) -> ("error out"=w539:errorcluster)
                      }
                    }
                    n537 = Select(t=w520, s=w525, f=u32 0) -> (s? t:f=w521:u32)
                    n538 = property on="Plane" class="DigNum (strict)"() -> ("Data Entry Limits"=w522:T13)  [unwired: 2 in, 2 out]
                    n539 = Bundle By Name(cluster=w522, "Maximum"=w521) -> (w515:T13)
                    n540 = property on="Plane" class="DigNum (strict)"("Data Entry Limits"=w515) -> ()  [unwired: 2 in, 2 out]
                  }
                  frame #1 {
                  }
                }
                n541 = call "HandleError.vi"("error in (no error)"=w512) -> ()
              }
            }
          }
          event #27 {
            n542 = event-data() -> ()  [unwired: 1 in, 1 out]
            n543 = property on="show position (PI digital)" class="Bool (strict)"() -> ("Value"=w543:bool)  [unwired: 2 in, 2 out]
            n544 = case shown="True" w543 {
              frame #0 {
                n545 = property on="Numeric" class="DigNum (strict)"("Visible"=FALSE) -> ()  [unwired: 2 in, 2 out]
                n546 = property on="Position" class="Arr (strict)"("Visible"=FALSE) -> ()  [unwired: 2 in, 2 out]
              }
              frame #1 {
                n547 = call "POS?.vi"("System no."=1, "All axes?"=TRUE) -> ("Position"=w546:dbl[])  [unwired: 16 in, 1 out]
                n548 = property on="Numeric" class="DigNum (strict)"("Visible"=TRUE) -> ()  [unwired: 2 in, 2 out]
                n549 = property on="Position" class="Arr (strict)"("Visible"=TRUE) -> ()  [unwired: 2 in, 2 out]
                n550 = local write "Position"(w546) -> ()
              }
            }
          }
          event #28 {
            n551 = event-data() -> ()  [unwired: 1 in, 5 out]
            n552 = local read "Display Settings"() -> (w551:T1)
            n553 = stacked-sequence {
              tunnel: w551 -> [_ w558 w564]
              frame #0 {
              }
              frame #1 {
                w553 = 0 ("index (vol)")
                n554 = call "ScannedImage.vi"() -> ("Scanned Image (output)"=w557:T11)  [unwired: 2 in]
                n555 = Unbundle By Name(w558) -> ("Plane"=w556:u32, "Threshold.max"=w555:u32)
                n556 = Unbundle By Name(w557) -> ("Trace"=w554:u32[][][][])
                n557 = call "ExtractImagePlane.vi"("Router"=w555, "Plane"=w556, "Trace"=w554) -> ()  [unwired: 1 out]
                n558 = local read "Image Settings"() -> (w559:T2)
                n559 = Index Array(array=w554, index (dim 0)=w553, index (dim 1)=w553) -> (element=w552:u32[][])  [unwired: 2 in]
                n560 = call "PickAndDestroy.vi"("Image Settings"=w559, "Threshold"=w555, "Image"=w552) -> ()
              }
              frame #2 {
                n561 = call "FIFOSettings.vi"() -> ("FIFO Settings(out)"=w562:T5)  [unwired: 2 in]
                n562 = call "UpdateFullImage.vi"("Display Settings"=w564) -> ()
                n563 = call "SPCSetParameters_HH.vi"("FIFO Settings"=w562) -> ("error (out)"=w563:errorcluster)  [unwired: 2 in]
                n564 = property class="VI"() -> ("VI Name"=w561:string)  [unwired: 2 in, 2 out]
                n565 = call "HandleError.vi"("error in (no error)"=w563) -> ()
                n566 = call "CallersName.vi"("Get/Set"=TRUE ("s"), "Callers Name"=w561) -> ()  [unwired: 1 out]
              }
            }
          }
          event #29 {
            n567 = event-data() -> ()  [unwired: 1 in, 5 out]
          }
          event #30 {
            n568 = event-data() -> ()  [unwired: 1 in, 6 out]
            n569 = call "AnalogSettings.vi"() -> ("Analog Settings (output)"=w568:T14)  [unwired: 2 in]
            n570 = call "AOTFSettings.vi"() -> ("AOTF Setting (Output)"=w569:T15)  [unwired: 2 in]
            n571 = Unbundle By Name(w569) -> ("Laser 1 Output Channel"=w566:tag, "AOTF  1 Output Voltage"=w565:dbl)
            n572 = Unbundle By Name(w568) -> ("PCI 671x Device Number"=w567:u32)
            n573 = case shown="True" "Laser 1" {
              tunnel: w567 -> [w572 w575]
              tunnel: w566 -> [w571 w576]
              tunnel: w565 -> [_ w574]
              frame #0 {
                n574 = call-poly "AO Update Channel (scaled value).vi"("value"=sgl 0.0, "channel (0)"=w571, "device"=w572) -> ()
              }
              frame #1 {
                n575 = call-poly "AO Update Channel (scaled value).vi"("value"=w574, "channel (0)"=w576, "device"=w575) -> ()
              }
            }
          }
          event #31 {
            n576 = event-data() -> ()  [unwired: 1 in, 6 out]
            n577 = call "AOTFSettings.vi"() -> ("AOTF Setting (Output)"=w582:T15)  [unwired: 2 in]
            n578 = call "AnalogSettings.vi"() -> ("Analog Settings (output)"=w581:T14)  [unwired: 2 in]
            n579 = Unbundle By Name(w582) -> ("Laser 2 Output Channel"=w579:tag, "AOTF  2 Output Voltage"=w578:dbl)
            n580 = Unbundle By Name(w581) -> ("PCI 671x Device Number"=w580:u32)
            n581 = case shown="False" "Laser 2" {
              tunnel: w580 -> [w584 w587]
              tunnel: w579 -> [w583 w588]
              tunnel: w578 -> [_ w586]
              frame #0 {
                n582 = call-poly "AO Update Channel (scaled value).vi"("value"=sgl 0.0, "channel (0)"=w583, "device"=w584) -> ()
              }
              frame #1 {
                n583 = call-poly "AO Update Channel (scaled value).vi"("value"=w586, "channel (0)"=w588, "device"=w587) -> ()
              }
            }
          }
          event #32 {
            n584 = event-data() -> ()  [unwired: 1 in, 6 out]
            n585 = call "AnalogSettings.vi"() -> ("Analog Settings (output)"=w593:T14)  [unwired: 2 in]
            n586 = call "AOTFSettings.vi"() -> ("AOTF Setting (Output)"=w594:T15)  [unwired: 2 in]
            n587 = Unbundle By Name(w594) -> ("Laser 3 Output Channel"=w591:tag, "AOTF  3 Output Voltage"=w590:dbl)
            n588 = Unbundle By Name(w593) -> ("PCI 671x Device Number"=w592:u32)
            n589 = case shown="True" "Laser 3" {
              tunnel: w592 -> [w596 w599]
              tunnel: w591 -> [w595 w600]
              tunnel: w590 -> [_ w598]
              frame #0 {
                n590 = call-poly "AO Update Channel (scaled value).vi"("value"=sgl 0.0, "channel (0)"=w595, "device"=w596) -> ()
              }
              frame #1 {
                n591 = call-poly "AO Update Channel (scaled value).vi"("value"=w598, "channel (0)"=w600, "device"=w599) -> ()
              }
            }
          }
          event #33 {
            n592 = event-data() -> ()  [unwired: 1 in, 6 out]
            n593 = call "AOTFSettings.vi"() -> ("AOTF Setting (Output)"=w606:T15)  [unwired: 2 in]
            n594 = call "AnalogSettings.vi"() -> ("Analog Settings (output)"=w605:T14)  [unwired: 2 in]
            n595 = Unbundle By Name(w606) -> ("Laser 4 Output Channel"=w603:tag, "AOTF  4 Output Voltage"=w602:dbl)
            n596 = Unbundle By Name(w605) -> ("PCI 671x Device Number"=w604:u32)
            n597 = case shown="True" "Laser 4" {
              tunnel: w604 -> [w608 w611]
              tunnel: w603 -> [w607 w612]
              tunnel: w602 -> [_ w610]
              frame #0 {
                n598 = call-poly "AO Update Channel (scaled value).vi"("value"=sgl 0.0, "channel (0)"=w607, "device"=w608) -> ()
              }
              frame #1 {
                n599 = call-poly "AO Update Channel (scaled value).vi"("value"=w610, "channel (0)"=w612, "device"=w611) -> ()
              }
            }
          }
          event #34 {
            n600 = event-data() -> ()  [unwired: 1 in, 6 out]
            n601 = call "AOTFSettings.vi"() -> ("AOTF Setting (Output)"=w618:T15)  [unwired: 2 in]
            n602 = call "AnalogSettings.vi"() -> ("Analog Settings (output)"=w617:T14)  [unwired: 2 in]
            n603 = Unbundle By Name(w618) -> ("Laser 5 Output Channel"=w615:tag, "AOTF 5 Output Voltage"=w614:dbl)
            n604 = Unbundle By Name(w617) -> ("PCI 671x Device Number"=w616:u32)
            n605 = case shown="True" "Laser 5" {
              tunnel: w616 -> [w620 w623]
              tunnel: w615 -> [w619 w624]
              tunnel: w614 -> [_ w622]
              frame #0 {
                n606 = call-poly "AO Update Channel (scaled value).vi"("value"=sgl 0.0, "channel (0)"=w619, "device"=w620) -> ()
              }
              frame #1 {
                n607 = call-poly "AO Update Channel (scaled value).vi"("value"=w622, "channel (0)"=w624, "device"=w623) -> ()
              }
            }
          }
          event #35 {
            n608 = event-data() -> ()  [unwired: 1 in, 6 out]
            n609 = call "AOTFSettings.vi"() -> ("AOTF Setting (Output)"=w630:T15)  [unwired: 2 in]
            n610 = call "AnalogSettings.vi"() -> ("Analog Settings (output)"=w629:T14)  [unwired: 2 in]
            n611 = Unbundle By Name(w630) -> ("Laser 6 Output Channel"=w627:tag, "AOTF  6 Output Voltage"=w626:dbl)
            n612 = Unbundle By Name(w629) -> ("PCI 671x Device Number"=w628:u32)
            n613 = case shown="True" "Laser 6" {
              tunnel: w628 -> [w632 w635]
              tunnel: w627 -> [w631 w636]
              tunnel: w626 -> [_ w634]
              frame #0 {
                n614 = call-poly "AO Update Channel (scaled value).vi"("value"=sgl 0.0, "channel (0)"=w631, "device"=w632) -> ()
              }
              frame #1 {
                n615 = call-poly "AO Update Channel (scaled value).vi"("value"=w634, "channel (0)"=w636, "device"=w635) -> ()
              }
            }
          }
          event #36 {
            n616 = event-data() -> ()  [unwired: 1 in, 6 out]
            n617 = call "AOTFSettings.vi"() -> ("AOTF Setting (Output)"=w642:T15)  [unwired: 2 in]
            n618 = call "AnalogSettings.vi"() -> ("Analog Settings (output)"=w641:T14)  [unwired: 2 in]
            n619 = Unbundle By Name(w642) -> ("Laser 7 Output Channel"=w639:tag, "AOTF 7 Output Voltage"=w638:dbl)
            n620 = Unbundle By Name(w641) -> ("PCI 671x Device Number"=w640:u32)
            n621 = case shown="True" "Laser 7" {
              tunnel: w640 -> [w644 w647]
              tunnel: w639 -> [w643 w648]
              tunnel: w638 -> [_ w646]
              frame #0 {
                n622 = call-poly "AO Update Channel.vi"("value"=sgl 0.0, "channel (0)"=w643, "device"=w644) -> ()
              }
              frame #1 {
                n623 = call-poly "AO Update Channel.vi"("value"=w646, "channel (0)"=w648, "device"=w647) -> ()
              }
            }
          }
          event #37 {
            n624 = event-data() -> ()  [unwired: 1 in, 6 out]
            n625 = call "AOTFSettings.vi"() -> ("AOTF Setting (Output)"=w654:T15)  [unwired: 2 in]
            n626 = call "AnalogSettings.vi"() -> ("Analog Settings (output)"=w653:T14)  [unwired: 2 in]
            n627 = Unbundle By Name(w654) -> ("Laser 8 Output Channel"=w651:tag, "AOTF  8 Output Voltage"=w650:dbl)
            n628 = Unbundle By Name(w653) -> ("PCI 671x Device Number"=w652:u32)
            n629 = case shown="True" "Laser 8" {
              tunnel: w652 -> [w656 w659]
              tunnel: w651 -> [w655 w660]
              tunnel: w650 -> [_ w658]
              frame #0 {
                n630 = call-poly "AO Update Channel.vi"("value"=sgl 0.0, "channel (0)"=w655, "device"=w656) -> ()
              }
              frame #1 {
                n631 = call-poly "AO Update Channel.vi"("value"=w658, "channel (0)"=w660, "device"=w659) -> ()
              }
            }
          }
        }
      }
    }
  }
